vi "PointGrey Grasshopper Temp_Cam.vi"(0 "Operation":T2(ring), 1 "Camera-specific in":variant, 5 "Exposure time (s)":dbl, 7 "Save path":path, 9 "Capture mode":enum16{"Single frame", "Sequence"}(ring), 11 "Capture button":refnum<vi>, 12 "Image in":variant, 14 "Frames in sequence":u32) -> (3 "Camera-specific out":variant, 4 "Status":T1)   [LabVIEW 2015]
uses:
  <vilib>/userdefined/High Color/IMAQdx.ctl
  <vilib>/vision/Image Controls.llb/IMAQ Image.ctl
  <vilib>/vision/driver/IMAQdx.llb/IMAQdx Camera Control Mode.ctl
  <vilib>/vision/driver/IMAQdx.llb/IMAQdx Acquisition Mode.ctl
  <vilib>/Platform/TimedLoop/XDataNode/timing_clust.ctl
  <vilib>/Platform/TimedLoop/XDataNode/nitl_modes.ctl
  <vilib>/Platform/TimedLoop/XDataNode/wakeup.ctl
  <vilib>/vision/driver/IMAQdx.llb/IMAQdx Buffer Number Mode.ctl
  <vilib>/platform/TimedLoop/XDataNode/XDataNode.xnode
  <vilib>/vision/driver/NI_Vision_Acquisition_Software.lvlib
  <resource>/objmgr/imaqdx.rc
  <vilib>/Platform/TimedLoop/XDataNode/XDNodeRunTimeDep.lvlib
  <vilib>/vision/NI_Vision_Development_Module.lvlib
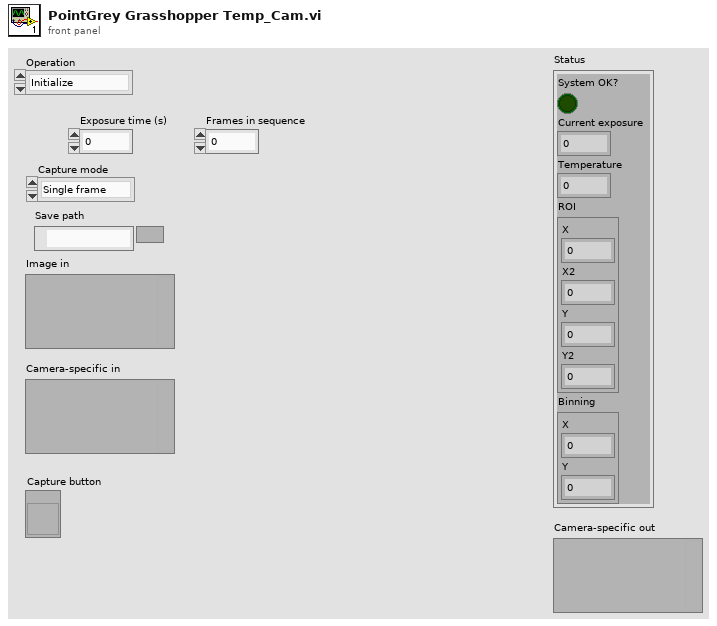
[diagram p1: front panel]
types:
  T1 = cluster{"System OK?":bool, "Current exposure":dbl, "Temperature":dbl, "ROI":cluster{"X":u32, "X2":u32, "Y":u32, "Y2":u32}, "Binning":cluster{"X":u32, "Y":u32}}
  T2 = enum16{"Initialize", "Shut down", "Set capture mode", "Set exposure", "Trigger and read", "Get status", "Other settings"}
  T3 = typedef "IMAQdx.ctl" = refnum<k21>
  T4 = typedef "IMAQ Image.ctl" = refnum<image>
  T5 = typedef "Semaphore RefNum" = refnum<k1>
  T6 = cluster{"Frames to capture":u32, "Current camera":i32, "Camera References":T3[], "Which cameras record":bool[], "Camera event refnums":refnum<event-registration>[], "Image buffers":T4[], "File write access":T5, "Offset and gain":dbl[][], "RGB Channels":enum16{"None", "Camera 1", "Camera 2", "Camera 3"}[], "RGB buffers":T4[], "Camera orientation":enum16{"No rotation, No flip", "No rotation, Flip UD", "No rotation, Flip LR", "Clockwise, No flip", "Clockwise, Flip UD", "Clockwise, Flip LR", "Anticlockwise, No flip", "Anticlockwise, Flip UD", "Anticlockwise, Flip LR"}[]}
  T7 = enum32{"Continuous", "Single frame", "Multi frame"}
  T8 = typedef "NI_Vision_Acquisition_Software.lvlib/IMAQdx Camera Control Mode.ctl" = enum32{"Controller", "Listener"}
  T9 = cluster{"New Image":T4, "Image":refnum<vi>, "FPS target":dbl}
  T10 = enum16{"open", "replace", "create", "open or create", "replace or create", "replace or create with confirmation"}
  T11 = cluster{"File refnum":refnum<file>, "Image File Directory":cluster{cluster{"Field":u16, "Type":u16, "Count":u32, "Value / Offset":u32, "Add IFD Offset?":bool}[], cluster{"Data":u32[], "Add offset?":bool}[]}, "Big endian?":bool, "IFD Offset Size":u32}
  T12 = typedef "NI_Vision_Acquisition_Software.lvlib/IMAQdx Acquisition Mode.ctl" = enum32{"One Shot", "Continuous"}
  T13 = typedef "XDNodeRunTimeDep.lvlib/timing_clust.ctl" = cluster{"Expected End [f-1]":u64, "Actual End [f-1]":u64, "Finished Late? [f-1]":bool, "Expected End [i-1]":u64, "Actual End [i-1]":u64, "Finished Late? [i-1]":bool, "Expected Start [i]":u64, "Actual Start [i]":u64, "Expected Start [f]":u64, "Actual Start [f]":u64, "Source Name":string, "Structure Name":string, "Period":i64, "Deadline":i64, "Offset":i64, "Start":i64, "Priority":i32, "Timeout":i32, "Mode":T14, "Wakeup Reason":T15, "Error":errorcluster, "Source Type":string, "Secondary Source Type":string, "Global End Time":u64, "Global Start Time":u64, "Frame Duration":u64, "Iteration Duration":u64, "Assigned CPU":i32, "I/O Scan Engine Mode":u32}
  T14 = typedef "XDNodeRunTimeDep.lvlib/nitl_modes.ctl" = enum32{"No Change", "Process missed periods, maintain original phase", "Discard missed periods, maintain original phase", "Process missed periods, ignore original phase", "Discard missed periods, ignore original phase"}
  T15 = typedef "XDNodeRunTimeDep.lvlib/wakeup.ctl" = enum32{"Normal", "Aborted", "Asynchronous wakeup", "Timing source error", "Timed loop error", "Timeout"}
  T16 = typedef "NI_Vision_Acquisition_Software.lvlib/IMAQdx Buffer Number Mode.ctl" = enum32{"Next", "Last", "Buffer Number", "Every", "Last New"}
  T17 = typedef "Image Type" = u32
  T18 = enum16{"No rotation, No flip", "No rotation, Flip UD", "No rotation, Flip LR", "Clockwise, No flip", "Clockwise, Flip UD", "Clockwise, Flip LR", "Anticlockwise, No flip", "Anticlockwise, Flip UD", "Anticlockwise, Flip LR"}[]
  T19 = enum16{"None", "Camera 1", "Camera 2", "Camera 3"}[]
  T20 = cluster{"Type":u32, "Version":u32, "Flags":u32, "SerialNumberHigh":u32, "SerialNumberLow":u32, "BusType":u32, "InterfaceName":string, "VendorName":string, "ModelName":string, "CameraFileName":string, "CameraAttributeURL":string}[]
  T21 = enum16{"None", "Camera 1", "Camera 2", "Camera 3"}
  T22 = cluster{"Camera identity":enum16{"Camera 1", "Camera 2", "Camera 3"}, "Timestamp":u64}
  T23 = enum16{"No rotation, No flip", "No rotation, Flip UD", "No rotation, Flip LR", "Clockwise, No flip", "Clockwise, Flip UD", "Clockwise, Flip LR", "Anticlockwise, No flip", "Anticlockwise, Flip UD", "Anticlockwise, Flip LR"}
  T24 = cluster{"element":enum16{"Camera 1", "Camera 2", "Camera 3"}, u64}
  T25 = cluster{"Camera identity":enum16{"Camera 1", "Camera 2", "Camera 3"}, "Timestamp":u64}[]
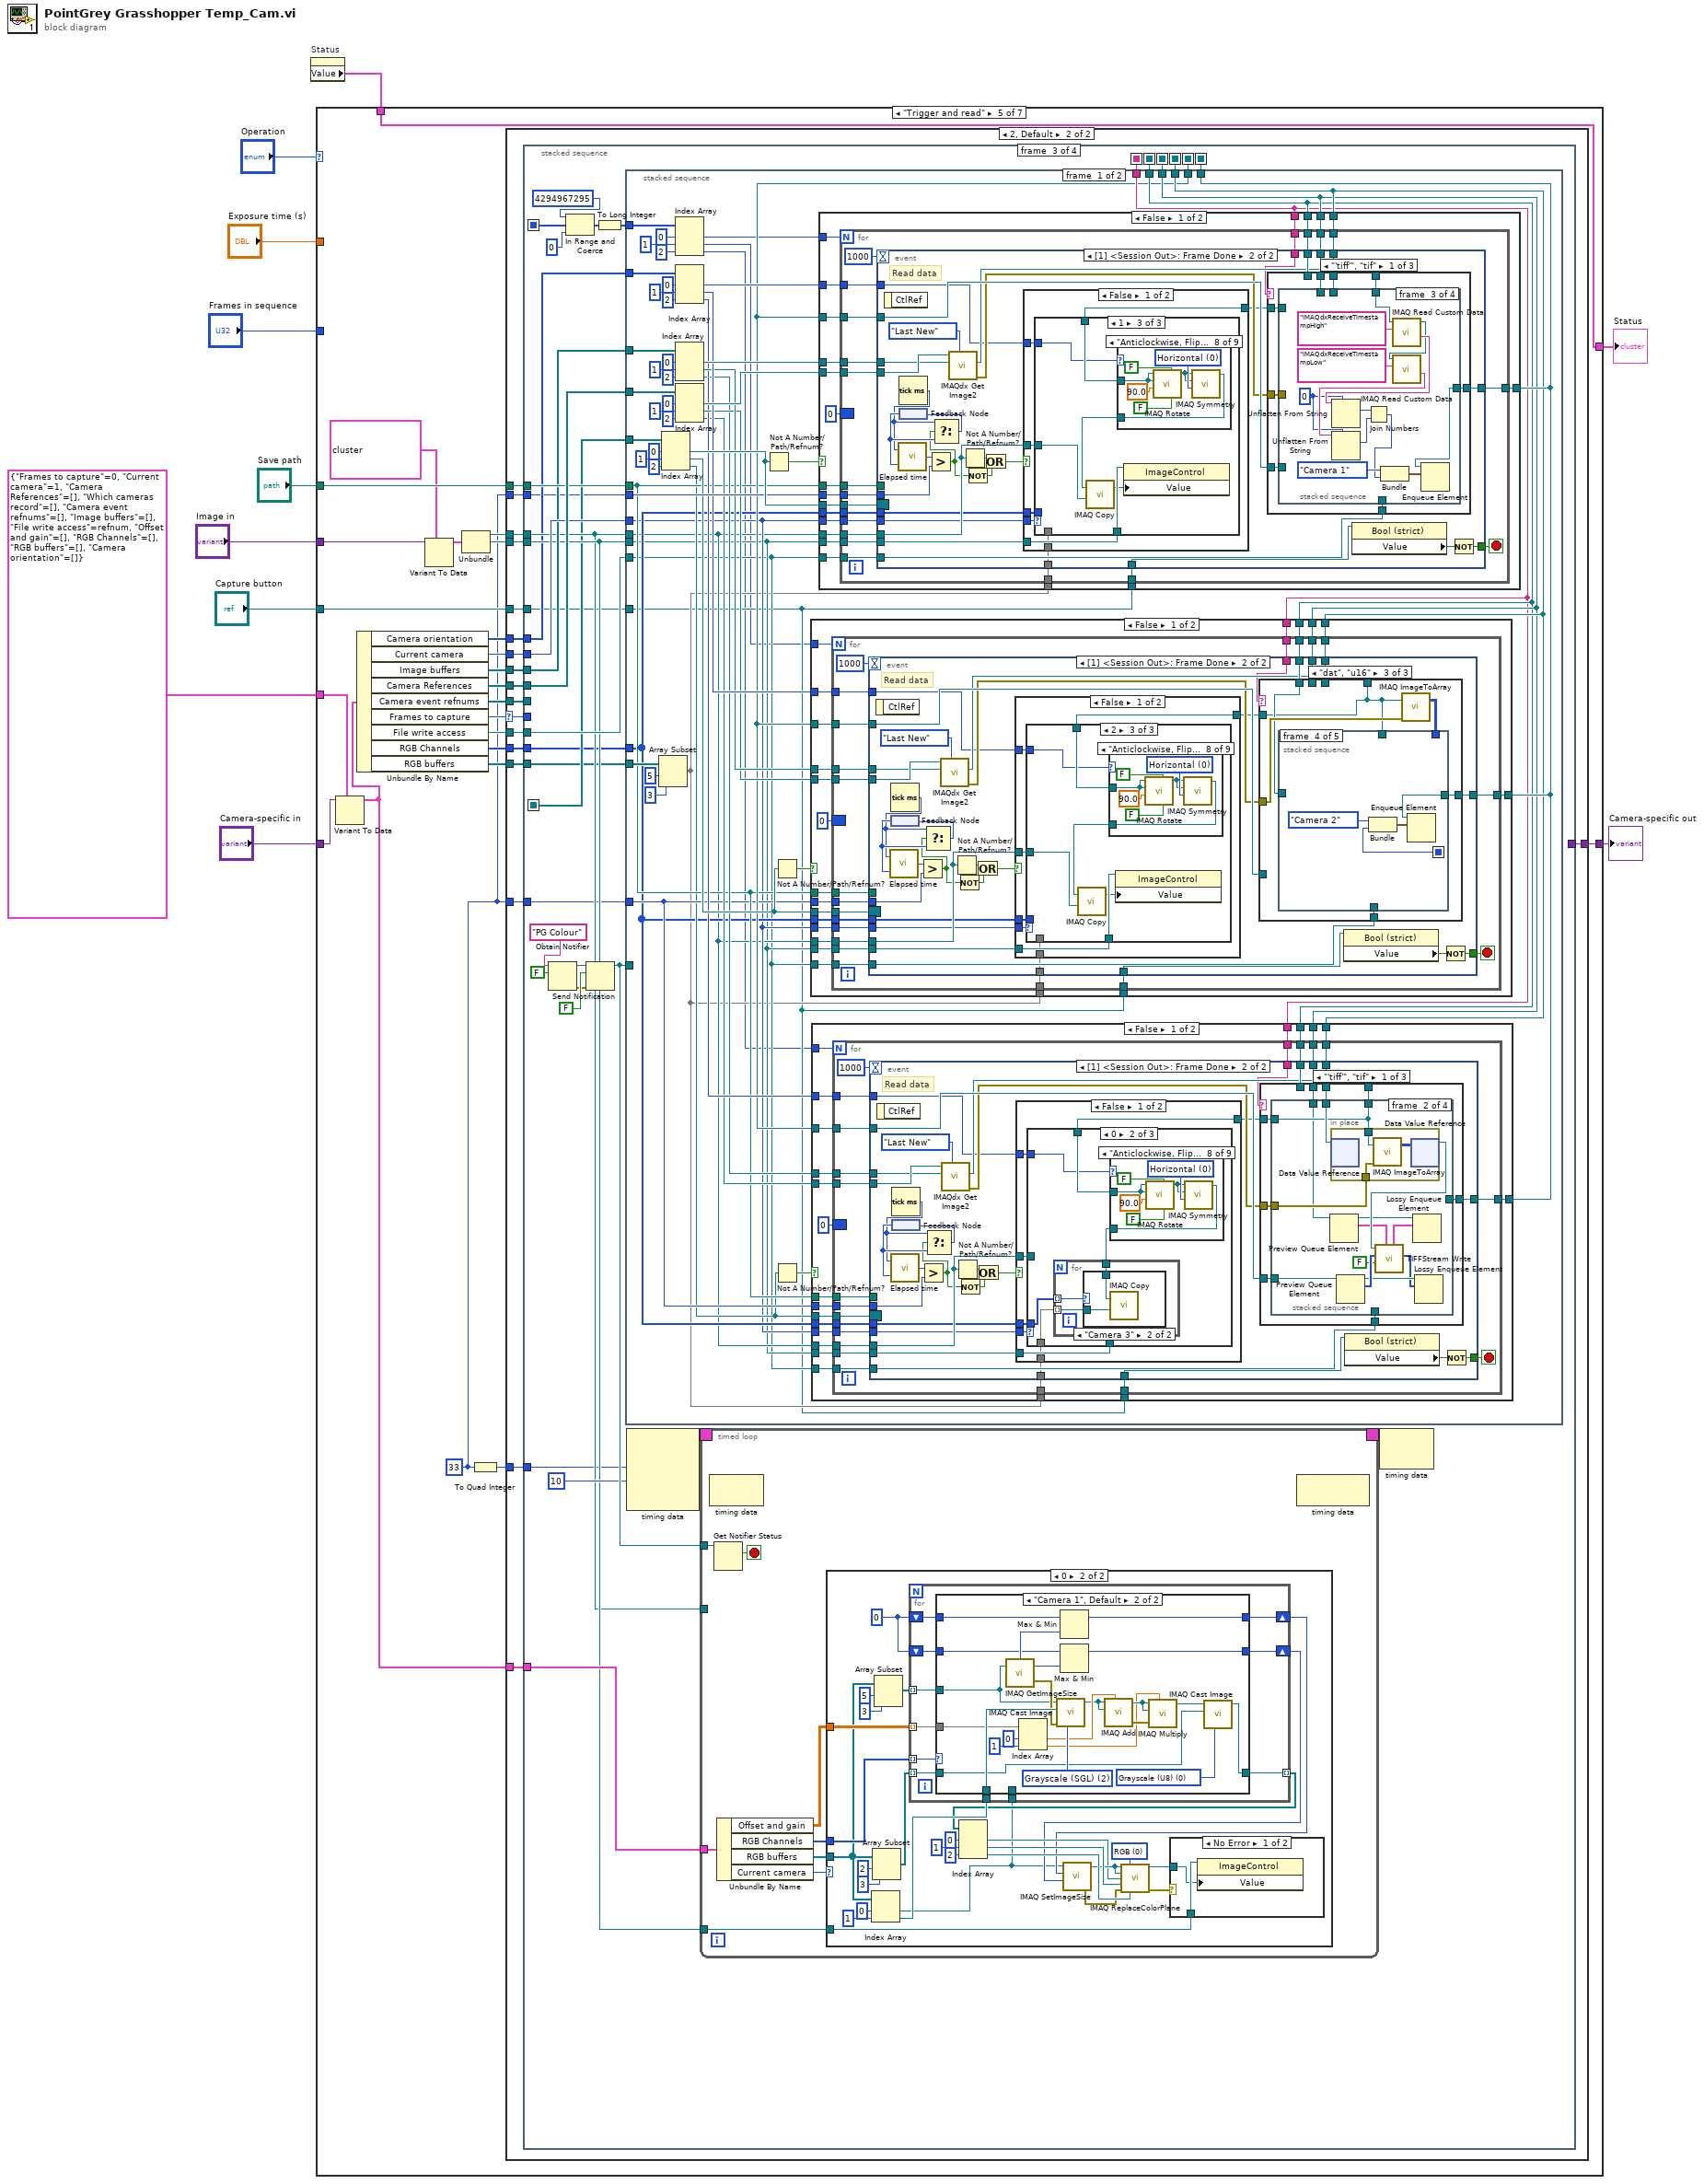
[diagram p0: block diagram]
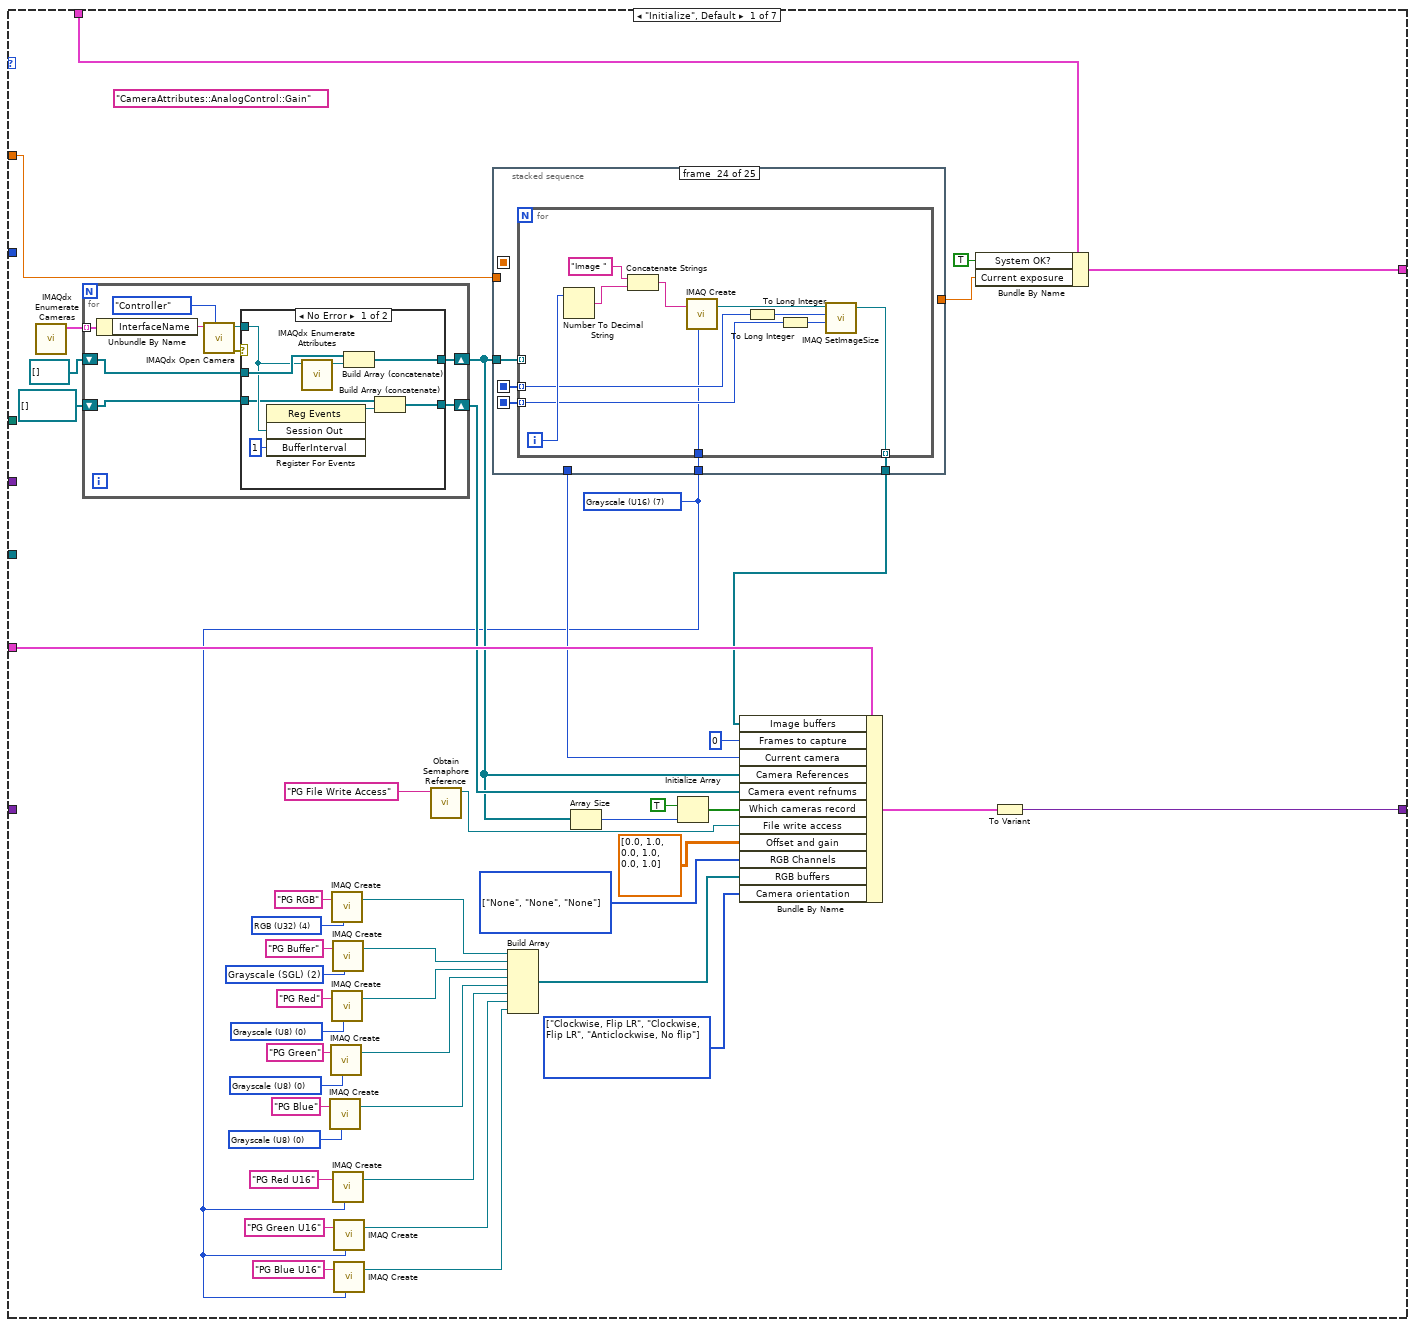
[diagram p2: hidden frame]
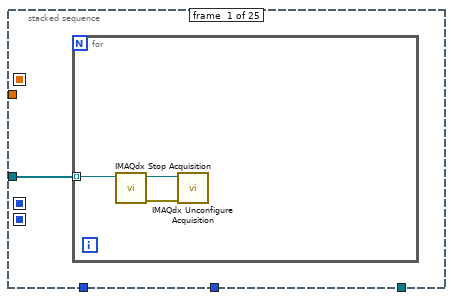
[diagram p3: hidden frame]
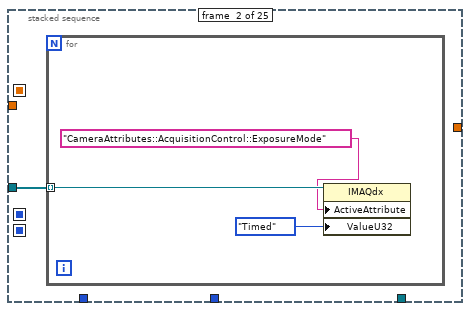
[diagram p4: hidden frame]
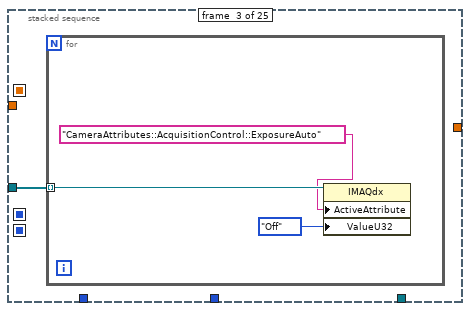
[diagram p5: hidden frame]
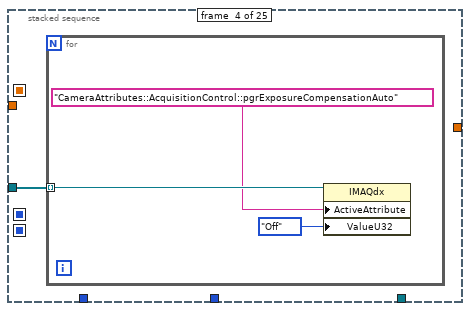
[diagram p6: hidden frame]
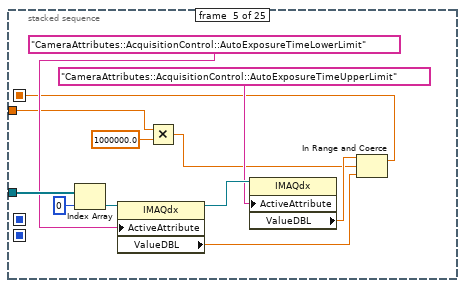
[diagram p7: hidden frame]
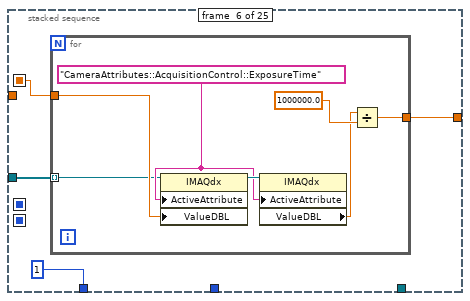
[diagram p8: hidden frame]
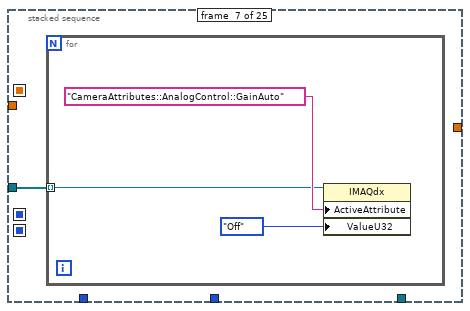
[diagram p9: hidden frame]
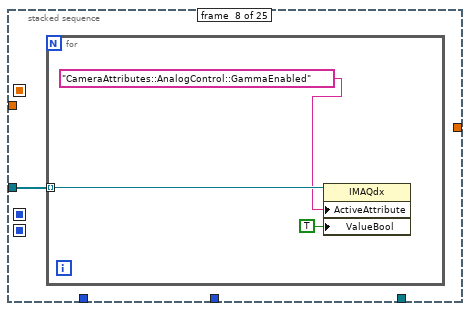
[diagram p10: hidden frame]
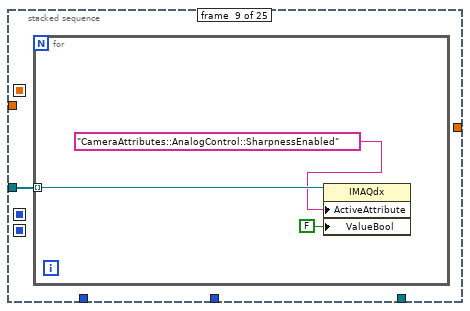
[diagram p11: hidden frame]
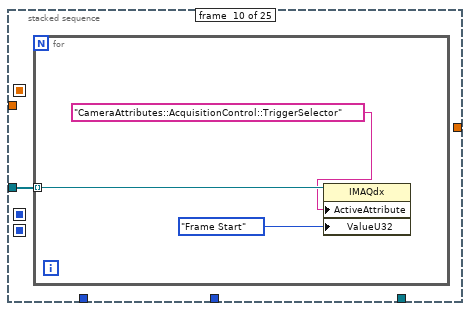
[diagram p12: hidden frame]
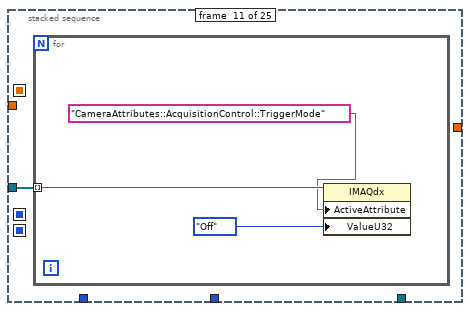
[diagram p13: hidden frame]
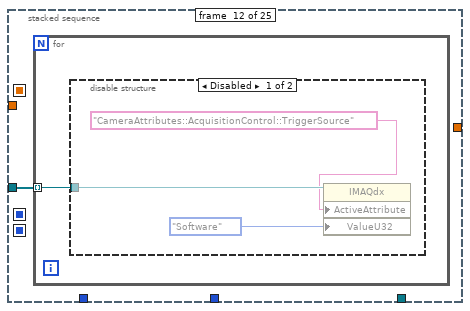
[diagram p14: hidden frame]
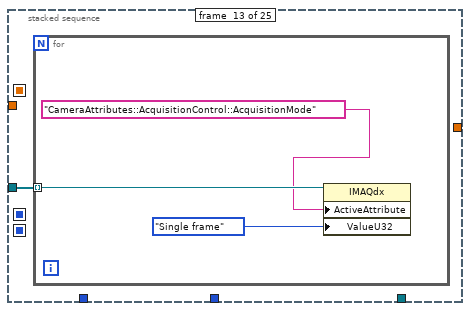
[diagram p16: hidden frame]
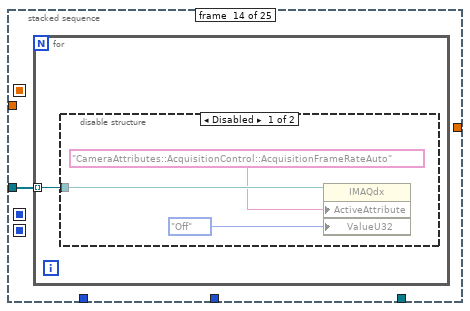
[diagram p17: hidden frame]
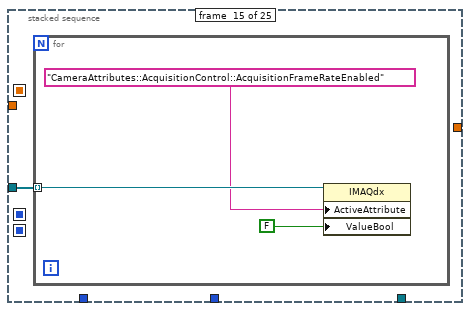
[diagram p19: hidden frame]
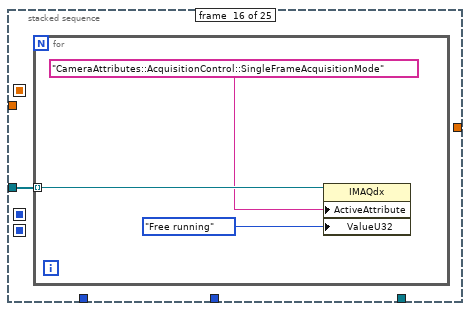
[diagram p20: hidden frame]
diagram:
  n1 = property on="Status" class="Clust (strict)"() -> ("Value"=w9:T1)  [unwired: 2 in, 2 out]
  n2 = case shown="\"Trigger and read\"" "Operation" {
    tunnel: "Exposure time (s)" -> [w47 _ _ w382 _ _ _]
    tunnel: w9 -> [w58 w218 w242 w388 w439 w1791 w1809]
    tunnel: [w57 w218 w242 w387 w439 w1790 w1809] -> w8
    tunnel: "Save path" -> [_ _ _ _ w438 _ _]
    tunnel: "Image in" -> [_ _ _ _ w429 _ _]
    tunnel: [w55 w213 w238 w385 w422 w1787 w1801] -> w5
    tunnel: "Camera-specific in" -> [_ w217 w240 w385 w425 w1787 w1808]
    tunnel: T6 {"Frames to capture"=0, "Current camera"=1, "Camera References"=[], "Which cameras record"=[], "Camera event refnums"=[], "Image buffers"=[], "File write access"=refnum, "Offset and gain"=[], "RGB Channels"=[], "RGB buffers"=[], "Camera orientation"=[]} -> [w56 w212 w239 w386 w437 w1786 w1807]
    tunnel: "Frames in sequence" -> [_ _ w235 _ _ _ _]
    tunnel: "Capture button" -> [_ _ _ _ w421 _ _]
    frame "Initialize", Default {
      w17 = T17 7 items=["Grayscale (U8)", "Grayscale (I16)", "Grayscale (SGL)", "Complex (CSG)", "RGB (U32)", "HSL (U32)", "RGB (U64)", "Grayscale (U16)"] ("Image Type")
      w19 = T18 [enum."Clockwise, Flip LR", enum."Clockwise, Flip LR", enum."Anticlockwise, No flip"] items=["No rotation, No flip", "No rotation, Flip UD", "No rotation, Flip LR", "Clockwise, No flip", "Clockwise, Flip UD", "Clockwise, Flip LR", "Anticlockwise, No flip", "Anticlockwise, Flip UD", "Anticlockwise, Flip LR"] ("Camera orientation")
      w26 = T17 0 items=["Grayscale (U8)", "Grayscale (I16)", "Grayscale (SGL)", "Complex (CSG)", "RGB (U32)", "HSL (U32)", "RGB (U64)", "Grayscale (U16)"] ("Image Type")
      w27 = T17 0 items=["Grayscale (U8)", "Grayscale (I16)", "Grayscale (SGL)", "Complex (CSG)", "RGB (U32)", "HSL (U32)", "RGB (U64)", "Grayscale (U16)"] ("Image Type")
      w28 = T17 0 items=["Grayscale (U8)", "Grayscale (I16)", "Grayscale (SGL)", "Complex (CSG)", "RGB (U32)", "HSL (U32)", "RGB (U64)", "Grayscale (U16)"] ("Image Type")
      w29 = T17 2 items=["Grayscale (U8)", "Grayscale (I16)", "Grayscale (SGL)", "Complex (CSG)", "RGB (U32)", "HSL (U32)", "RGB (U64)", "Grayscale (U16)"] ("Image Type")
      w30 = T17 4 items=["Grayscale (U8)", "Grayscale (I16)", "Grayscale (SGL)", "Complex (CSG)", "RGB (U32)", "HSL (U32)", "RGB (U64)", "Grayscale (U16)"] ("Image Type")
      w36 = T19 [enum."None", enum."None", enum."None"] items=["None", "Camera 1", "Camera 2", "Camera 3"] ("RGB Channels")
      (unwired) "CameraAttributes::AnalogControl::Gain"
      n3 = call <vilib>:"IMAQdx Enumerate Cameras.vi"() -> ("Camera Information Array"=w53:T20)  [unwired: 10 in, 1 out]
      n4 = for {
        tunnel: w53 -> [w198] mode=indexing
        shift-right: [w193] -> w45
        shift-left: T3[] [] -> [w191]
        shift-right: [w194] -> w50
        shift-left: refnum<event-registration>[] [] -> [w190]
        n5 = Unbundle By Name(w198) -> ("InterfaceName"=w197:string)
        n6 = call <vilib>:"IMAQdx Open Camera.vi"("Camera Control Mode"=IMAQdx_Camera_Control_Mode."Controller", "Session In"=w197) -> ("error out"=w192:errorcluster, "Session Out"=w195:T3)  [unwired: 8 in]
        n7 = case shown="No Error" w192 {
          tunnel: w195 -> [w202 _]
          tunnel: [w201 w207] -> w194
          tunnel: [w204 w208] -> w193
          tunnel: w191 -> [w203 w208]
          tunnel: w190 -> [w199 w207]
          frame No Error {
            n8 = register-events(w202, u32 1 ("BufferInterval")) -> (reference out=w200:refnum<event-registration>)  [unwired: 2 in, 1 out]
            n9 = call <vilib>:"IMAQdx Enumerate Attributes.vi"("Session In"=w202) -> ("Session Out"=w205:T3)  [unwired: 8 in, 2 out]
            n10 = Build Array (concatenate)(w203, w205) -> (w204:T3[])
            n11 = Build Array (concatenate)(w199, w200) -> (w201:refnum<event-registration>[])
          }
          frame Error {
          }
        }
      }
      n12 = call "IMAQ Create"("Image Name"="PG Blue", "Image Type"=w26) -> ("New Image"=w21:T4)  [unwired: 3 in, 1 out]
      n13 = call "IMAQ Create"("Image Name"="PG Green", "Image Type"=w27) -> ("New Image"=w22:T4)  [unwired: 3 in, 1 out]
      n14 = call "IMAQ Create"("Image Name"="PG RGB", "Image Type"=w30) -> ("New Image"=w25:T4)  [unwired: 3 in, 1 out]
      n15 = call "IMAQ Create"("Image Name"="PG Red", "Image Type"=w28) -> ("New Image"=w23:T4)  [unwired: 3 in, 1 out]
      n16 = call "IMAQ Create"("Image Name"="PG Buffer", "Image Type"=w29) -> ("New Image"=w24:T4)  [unwired: 3 in, 1 out]
      n17 = call "IMAQ Create"("Image Name"="PG Red U16", "Image Type"=w17) -> ("New Image"=w16:T4)  [unwired: 3 in, 1 out]
      n18 = call "IMAQ Create"("Image Name"="PG Green U16", "Image Type"=w17) -> ("New Image"=w14:T4)  [unwired: 3 in, 1 out]
      n19 = call "IMAQ Create"("Image Name"="PG Blue U16", "Image Type"=w17) -> ("New Image"=w15:T4)  [unwired: 3 in, 1 out]
      n20 = call <vilib>:"Obtain Semaphore Reference.vi"("name (unnamed)"="PG File Write Access") -> ("semaphore"=w38:T5)  [unwired: 4 in, 2 out]
      n21 = stacked-sequence {
        seq-local: [_ _ _ _ w78 _ _ _ _ _ _ _ _ _ _ _ _ _ _ _ _ _ _ _ _] -> [_ _ _ _ _ w87 _ _ _ _ _ _ _ _ _ _ _ _ _ _ _ _ _ _ _]
        seq-local: [_ _ _ _ _ _ _ _ _ _ _ _ _ _ _ _ _ w144 _ _ _ _ _ _ _] -> [_ _ _ _ _ _ _ _ _ _ _ _ _ _ _ _ _ _ _ _ _ _ _ w175 _]
        seq-local: [_ _ _ _ _ _ _ _ _ _ _ _ _ _ _ _ _ _ w150 _ _ _ _ _ _] -> [_ _ _ _ _ _ _ _ _ _ _ _ _ _ _ _ _ _ _ _ _ _ _ w174 _]
        tunnel: w45 -> [w59 w63 w67 w71 w84 w90 w98 w102 w106 w110 w114 w118 w123 w127 w132 w136 w140 w145 w151 w156 w160 w164 w168 w176 w188]
        tunnel: [_ _ _ _ _ 1 ("index") _ _ _ _ _ _ _ _ _ _ _ _ _ _ _ _ _ _ _] -> w48
        tunnel: w47 -> [_ _ _ _ w76 _ _ _ _ _ _ _ _ _ _ _ _ _ _ _ _ _ _ _ _]
        tunnel: [_ _ _ _ _ w88 _ _ _ _ _ _ _ _ _ _ _ _ _ _ _ _ _ _ _] -> w46
        tunnel: [_ _ _ _ _ _ _ _ _ _ _ _ _ _ _ _ _ _ _ _ _ _ _ w173 _] -> w41
        tunnel: w17 -> [_ _ _ _ _ _ _ _ _ _ _ _ _ _ _ _ _ _ _ _ _ _ _ w172 _]
        frame #0 {
          n22 = for {
            tunnel: w59 -> [w62] mode=indexing
            n23 = call <vilib>:"IMAQdx Stop Acquisition.vi"("Session In"=w62) -> ("error out"=w60:errorcluster, "Session Out"=w61:T3)  [unwired: 9 in]
            n24 = call <vilib>:"IMAQdx Unconfigure Acquisition.vi"("error in"=w60, "Session In"=w61) -> ()  [unwired: 8 in, 2 out]
          }
        }
        frame #1 {
          n25 = for {
            tunnel: w63 -> [w66] mode=indexing
            n26 = property class="IMAQdx"(reference=w66, "ActiveAttribute"="CameraAttributes::AcquisitionControl::ExposureMode", "ValueU32"=enum32{"Timed", "Trigger Width"}."Timed") -> ()  [unwired: 1 in, 2 out]
          }
        }
        frame #2 {
          n27 = for {
            tunnel: w67 -> [w70] mode=indexing
            n28 = property class="IMAQdx"(reference=w70, "ActiveAttribute"="CameraAttributes::AcquisitionControl::ExposureAuto", "ValueU32"=enum32{"Off", "Once", "Continuous"}."Off") -> ()  [unwired: 1 in, 2 out]
          }
        }
        frame #3 {
          n29 = for {
            tunnel: w71 -> [w74] mode=indexing
            n30 = property class="IMAQdx"(reference=w74, "ActiveAttribute"="CameraAttributes::AcquisitionControl::pgrExposureCompensationAuto", "ValueU32"=enum32{"Off", "Once", "Continuous"}."Off") -> ()  [unwired: 1 in, 2 out]
          }
        }
        frame #4 {
          n31 = Index Array(array=w84, index=0) -> (element=w86:T3)
          n32 = property class="IMAQdx"(reference=w86, "ActiveAttribute"="CameraAttributes::AcquisitionControl::AutoExposureTimeLowerLimit") -> (reference out=w82:T3, "ValueDBL"=w80:dbl)  [unwired: 1 in, 1 out]
          n33 = Multiply(x=w76, y=1000000.0) -> (x*y=w75:dbl)
          n34 = property class="IMAQdx"(reference=w82, "ActiveAttribute"="CameraAttributes::AcquisitionControl::AutoExposureTimeUpperLimit") -> ("ValueDBL"=w79:dbl)  [unwired: 1 in, 2 out]
          n35 = In Range and Coerce(upper limit=w79, x=w75, lower limit=w80) -> (coerced(x)=w78:dbl)  [unwired: 1 out]
        }
        frame #5 {
          n36 = for {
            tunnel: w90 -> [w91] mode=indexing
            tunnel: [w94] -> w88
            tunnel: w87 -> [w92]
            w93 = "CameraAttributes::AcquisitionControl::ExposureTime"
            n37 = property class="IMAQdx"(reference=w91, "ActiveAttribute"=w93, "ValueDBL"=w92) -> (reference out=w97:T3)  [unwired: 1 in, 1 out]
            n38 = property class="IMAQdx"(reference=w97, "ActiveAttribute"=w93) -> ("ValueDBL"=w95:dbl)  [unwired: 1 in, 2 out]
            n39 = Divide(x=w95, y=1000000.0) -> (x/y=w94:dbl)
          }
        }
        frame #6 {
          n40 = for {
            tunnel: w98 -> [w99] mode=indexing
            n41 = property class="IMAQdx"(reference=w99, "ActiveAttribute"="CameraAttributes::AnalogControl::GainAuto", "ValueU32"=enum32{"Off", "Once", "Continuous"}."Off") -> ()  [unwired: 1 in, 2 out]
          }
        }
        frame #7 {
          n42 = for {
            tunnel: w102 -> [w105] mode=indexing
            n43 = property class="IMAQdx"(reference=w105, "ActiveAttribute"="CameraAttributes::AnalogControl::GammaEnabled", "ValueBool"=TRUE) -> ()  [unwired: 1 in, 2 out]
          }
        }
        frame #8 {
          n44 = for {
            tunnel: w106 -> [w109] mode=indexing
            n45 = property class="IMAQdx"(reference=w109, "ActiveAttribute"="CameraAttributes::AnalogControl::SharpnessEnabled", "ValueBool"=FALSE) -> ()  [unwired: 1 in, 2 out]
          }
        }
        frame #9 {
          n46 = for {
            tunnel: w110 -> [w113] mode=indexing
            n47 = property class="IMAQdx"(reference=w113, "ActiveAttribute"="CameraAttributes::AcquisitionControl::TriggerSelector", "ValueU32"=enum32{"Frame Start", "Exposure Active"}."Frame Start") -> ()  [unwired: 1 in, 2 out]
          }
        }
        frame #10 {
          n48 = for {
            tunnel: w114 -> [w117] mode=indexing
            n49 = property class="IMAQdx"(reference=w117, "ActiveAttribute"="CameraAttributes::AcquisitionControl::TriggerMode", "ValueU32"=enum32{"Off", "On"}."Off") -> ()  [unwired: 1 in, 2 out]
          }
        }
        frame #11 {
          n50 = for {
            tunnel: w118 -> [w119] mode=indexing
            n51 = disable-structure shown="Disabled" {
              disable-tunnel: w119 -> [w122 _]
              frame Disabled {
                n52 = property class="IMAQdx"(reference=w122, "ActiveAttribute"="CameraAttributes::AcquisitionControl::TriggerSource", "ValueU32"=enum32{"Software", "Line 0", "Line 2", "Line 3"}."Software") -> ()  [unwired: 1 in, 2 out]
              }
              frame Enabled {
              }
            }
          }
        }
        frame #12 {
          n53 = for {
            tunnel: w123 -> [w126] mode=indexing
            n54 = property class="IMAQdx"(reference=w126, "ActiveAttribute"="CameraAttributes::AcquisitionControl::AcquisitionMode", "ValueU32"=T7."Single frame") -> ()  [unwired: 1 in, 2 out]
          }
        }
        frame #13 {
          n55 = for {
            tunnel: w127 -> [w128] mode=indexing
            n56 = disable-structure shown="Disabled" {
              disable-tunnel: w128 -> [w131 _]
              frame Disabled {
                n57 = property class="IMAQdx"(reference=w131, "ActiveAttribute"="CameraAttributes::AcquisitionControl::AcquisitionFrameRateAuto", "ValueU32"=enum32{"Off", "Continuous"}."Off") -> ()  [unwired: 1 in, 2 out]
              }
              frame Enabled {
              }
            }
          }
        }
        frame #14 {
          n58 = for {
            tunnel: w132 -> [w135] mode=indexing
            n59 = property class="IMAQdx"(reference=w135, "ActiveAttribute"="CameraAttributes::AcquisitionControl::AcquisitionFrameRateEnabled", "ValueBool"=FALSE) -> ()  [unwired: 1 in, 2 out]
          }
        }
        frame #15 {
          n60 = for {
            tunnel: w136 -> [w139] mode=indexing
            n61 = property class="IMAQdx"(reference=w139, "ActiveAttribute"="CameraAttributes::AcquisitionControl::SingleFrameAcquisitionMode", "ValueU32"=enum16{"Free running", "Triggered"}."Free running") -> ()  [unwired: 1 in, 2 out]
          }
        }
        frame #16 {
          n62 = for {
            tunnel: w140 -> [w143] mode=indexing
            w142 = u32 17563654 items=["Mono 8"=17301505, "Mono 12 Packed (IIDC-msb)"=17563654, "Mono 12 Packed"=17563719, "Mono 16"=17825799]
            n63 = property class="IMAQdx"(reference=w143, "ActiveAttribute"="CameraAttributes::ImageFormatControl::PixelFormat", "ValueU32"=w142) -> ()  [unwired: 1 in, 2 out]
          }
        }
        frame #17 {
          n64 = for {
            tunnel: w145 -> [w149] mode=indexing
            tunnel: [w146] -> w144 mode=indexing
            w148 = "CameraAttributes::ImageFormatControl::Width"
            n65 = property class="IMAQdx"(reference=w149, "ActiveAttribute"=w148) -> (reference out=w147:T3, "MaxU32"=w146:u32)  [unwired: 1 in, 1 out]
            n66 = property class="IMAQdx"(reference=w147, "ActiveAttribute"=w148, "ValueU32"=w146) -> ()  [unwired: 1 in, 2 out]
          }
        }
        frame #18 {
          n67 = for {
            tunnel: w151 -> [w155] mode=indexing
            tunnel: [w152] -> w150 mode=indexing
            w154 = "CameraAttributes::ImageFormatControl::Height"
            n68 = property class="IMAQdx"(reference=w155, "ActiveAttribute"=w154) -> (reference out=w153:T3, "MaxU32"=w152:u32)  [unwired: 1 in, 1 out]
            n69 = property class="IMAQdx"(reference=w153, "ActiveAttribute"=w154, "ValueU32"=w152) -> ()  [unwired: 1 in, 2 out]
          }
        }
        frame #19 {
          n70 = for {
            tunnel: w156 -> [w158] mode=indexing
            n71 = property class="IMAQdx"(reference=w158, "ActiveAttribute"="CameraAttributes::ImageFormatControl::OffsetX", "ValueU32"=u32 0) -> ()  [unwired: 1 in, 2 out]
          }
        }
        frame #20 {
          n72 = for {
            tunnel: w160 -> [w162] mode=indexing
            n73 = property class="IMAQdx"(reference=w162, "ActiveAttribute"="CameraAttributes::ImageFormatControl::OffsetY", "ValueU32"=u32 0) -> ()  [unwired: 1 in, 2 out]
          }
        }
        frame #21 {
          n74 = for {
            tunnel: w164 -> [w166] mode=indexing
            n75 = property class="IMAQdx"(reference=w166, "ActiveAttribute"="CameraAttributes::ImageFormatControl::BinningVertical", "ValueU32"=u32 1) -> ()  [unwired: 1 in, 2 out]
          }
        }
        frame #22 {
          n76 = for {
            tunnel: w168 -> [w170] mode=indexing
            w169 = u16 7 items=["Standard"=0, "2x2 Binning"=1, "2x2 Decimation"=2, "High sensitivity 12-bit ADC"=7]
            n77 = property class="IMAQdx"(reference=w170, "ActiveAttribute"="CameraAttributes::ImageFormatControl::VideoMode", "ValueU32"=w169) -> ()  [unwired: 1 in, 2 out]
          }
        }
        frame #23 {
          n78 = for {
            tunnel: w176 -> [_] mode=indexing
            tunnel: w175 -> [w181] mode=indexing
            tunnel: w174 -> [w180] mode=indexing
            tunnel: [w182] -> w173 mode=indexing
            tunnel: w172 -> [w177]
            i -> [w186]
            n79 = Number To Decimal String(number=w186) -> (decimal integer string=w185:string)  [unwired: 1 in]
            n80 = Concatenate Strings("Image ", w185) -> (w184:string)
            n81 = call "IMAQ Create"("Image Name"=w184, "Image Type"=w177) -> ("New Image"=w183:T4)  [unwired: 3 in, 1 out]
            n82 = To Long Integer(number=w181) -> (32bit integer=w179:i32)
            n83 = To Long Integer(number=w180) -> (32bit integer=w178:i32)
            n84 = call "IMAQ SetImageSize"("Y Resolution"=w178, "X Resolution"=w179, "Image"=w183) -> ("Image Out"=w182:T4)  [unwired: 2 in, 1 out]
          }
        }
        frame #24 {
          n85 = for {
            tunnel: w188 -> [w189] mode=indexing
            n86 = call <vilib>:"IMAQdx Configure Grab.vi"("Session In"=w189) -> ()  [unwired: 9 in, 2 out]
          }
        }
      }
      n87 = Build Array(w25, w24, w23, w22, w21, w16, w14, w15) -> (w20:T4[])
      n88 = Array Size(array=w45) -> (size(s)=w43:i32)
      n89 = Initialize Array(TRUE, w43) -> (w42:bool[])
      n90 = Bundle By Name(cluster=w56, "Image buffers"=w41, "Frames to capture"=u32 0, "Current camera"=w48, "Camera References"=w45, "Camera event refnums"=w50, "Which cameras record"=w42, "File write access"=w38, "Offset and gain"=dbl[][] [[0.0, 1.0], [0.0, 1.0], [0.0, 1.0]], "RGB Channels"=w36, "RGB buffers"=w20, "Camera orientation"=w19) -> (w51:T6)
      n91 = Bundle By Name(cluster=w58, "System OK?"=TRUE, "Current exposure"=w46) -> (w57:T1)
      n92 = To Variant(anything=w51) -> (Variant=w55:variant)
    }
    frame "Shut down" {
      n93 = Variant To Data(type=w212, Variant=w217) -> (data=w216:T6)  [unwired: 1 in, 1 out]
      n94 = Unbundle By Name(w216) -> ("Camera References"=w215:T3[], "Camera event refnums"=w214:refnum<event-registration>[], "File write access"=w211:T5, "Image buffers"=w210:T4[], "RGB buffers"=w209:T4[])
      n95 = for {
        tunnel: w210 -> [w220] mode=indexing
        n96 = call "IMAQ Dispose"("Image"=w220) -> ()  [unwired: 5 in, 1 out]
      }
      n97 = for {
        tunnel: w209 -> [w219] mode=indexing
        n98 = call "IMAQ Dispose"("Image"=w219) -> ()  [unwired: 5 in, 1 out]
      }
      n99 = stacked-sequence {
        tunnel: w215 -> [w221 _]
        tunnel: w214 -> [_ w227]
        frame #0 {
          n100 = for {
            tunnel: w221 -> [w222] mode=indexing
            n101 = call <vilib>:"IMAQdx Stop Acquisition.vi"("Session In"=w222) -> ("error out"=w226:errorcluster, "Session Out"=w225:T3)  [unwired: 9 in]
            n102 = call <vilib>:"IMAQdx Unconfigure Acquisition.vi"("error in"=w226, "Session In"=w225) -> ("error out"=w224:errorcluster, "Session Out"=w223:T3)  [unwired: 8 in]
            n103 = call <vilib>:"IMAQdx Close Camera.vi"("error in"=w224, "Session In"=w223) -> ()  [unwired: 9 in, 1 out]
          }
        }
        frame #1 {
          n104 = for {
            tunnel: w227 -> [w229] mode=indexing
            n105 = Unregister For Events(event registration refnum=w229) -> (error out=w228:errorcluster)  [unwired: 1 in]
            n106 = call <vilib>:"Clear Errors.vi"("error in (no error)"=w228) -> ()  [unwired: 5 in, 2 out]
          }
        }
      }
      n107 = call <vilib>:"Release Semaphore Reference.vi"("semaphore"=w211) -> ()  [unwired: 9 in, 2 out]
      n108 = To Variant(anything=w212) -> (Variant=w213:variant)
    }
    frame "Set capture mode" {
      n109 = Variant To Data(type=w239, Variant=w240) -> (data=w234:T6)  [unwired: 1 in, 1 out]
      n110 = Unbundle By Name(w234) -> ("Camera References"=w233:T3[], "Camera event refnums"=w231:refnum<event-registration>[], "Which cameras record"=w232:bool[])
      n111 = case shown="\"Sequence\"" "Capture mode" {
        tunnel: [w243 w313] -> w236
        tunnel: w235 -> [w244 w314]
        tunnel: w233 -> [w248 w318]
        tunnel: w232 -> [w247 w317]
        tunnel: w231 -> [w246 w316]
        tunnel: [w245 w315] -> w230
        frame "Sequence" {
          n112 = stacked-sequence {
            tunnel: w248 -> [_ w257]
            tunnel: w247 -> [_ w256]
            tunnel: w246 -> [w250 w253]
            tunnel: [_ w255] -> w245
            tunnel: w244 -> [w249 w254]
            tunnel: [w249 _] -> w243
            frame #0 {
              n113 = disable-structure shown="Enabled" {
                disable-tunnel: w250 -> [w251 _]
                frame Disabled {
                  n114 = for {
                    tunnel: w251 -> [w252] mode=indexing
                    n115 = Unregister For Events(event registration refnum=w252) -> ()  [unwired: 1 in, 1 out]
                  }
                }
                frame Enabled {
                }
              }
            }
            frame #1 {
              n116 = for {
                tunnel: w257 -> [w262] mode=indexing
                tunnel: w256 -> [w263] mode=indexing
                shift-right: [w261] -> w255
                shift-left: w253 -> [w260]
                tunnel: w254 -> [w259]
                i -> [w258]
                n117 = case shown="True" w263 {
                  tunnel: w262 -> [_ w267]
                  tunnel: [w264 w268] -> w261
                  tunnel: w260 -> [w264 w269]
                  tunnel: w259 -> [_ w266]
                  tunnel: w258 -> [_ w265]
                  frame False {
                  }
                  frame True {
                    n118 = stacked-sequence {
                      tunnel: w269 -> [_ _ _ _ _ _ _ _ w300 _]
                      tunnel: [_ _ _ _ _ _ _ _ w301 _] -> w268
                      tunnel: w267 -> [w272 w273 w281 w285 w288 w292 w294 w297 w302 w310]
                      tunnel: w266 -> [_ _ w280 _ _ _ _ _ _ _]
                      tunnel: w265 -> [_ _ _ _ _ _ _ _ w299 _]
                      frame #0 {
                        n119 = call <vilib>:"IMAQdx Stop Acquisition.vi"("Session In"=w272) -> ("error out"=w270:errorcluster, "Session Out"=w271:T3)  [unwired: 9 in]
                        n120 = call <vilib>:"IMAQdx Unconfigure Acquisition.vi"("error in"=w270, "Session In"=w271) -> ()  [unwired: 8 in, 2 out]
                      }
                      frame #1 {
                        n121 = disable-structure shown="Enabled" {
                          disable-tunnel: w273 -> [w274 w277]
                          frame Disabled {
                            n122 = property class="IMAQdx"(reference=w274, "ActiveAttribute"="CameraAttributes::AcquisitionControl::AcquisitionMode", "ValueU32"=T7."Multi frame") -> ()  [unwired: 1 in, 2 out]
                          }
                          frame Enabled {
                            n123 = property class="IMAQdx"(reference=w277, "ActiveAttribute"="CameraAttributes::AcquisitionControl::AcquisitionMode", "ValueU32"=T7."Continuous") -> ()  [unwired: 1 in, 2 out]
                          }
                        }
                      }
                      frame #2 {
                        n124 = disable-structure shown="Enabled" {
                          disable-tunnel: w281 -> [w283 _]
                          disable-tunnel: w280 -> [w282 _]
                          frame Disabled {
                            n125 = property class="IMAQdx"(reference=w283, "ActiveAttribute"="CameraAttributes::AcquisitionControl::AcquisitionFrameCount", "ValueU32"=w282) -> ()  [unwired: 1 in, 2 out]
                          }
                          frame Enabled {
                          }
                        }
                      }
                      frame #3 {
                        n126 = property class="IMAQdx"(reference=w285, "ActiveAttribute"="CameraAttributes::AcquisitionControl::TriggerSource", "ValueU32"=enum32{"Software", "Line 0", "Line 2", "Line 3"}."Software") -> ()  [unwired: 1 in, 2 out]
                      }
                      frame #4 {
                        n127 = property class="IMAQdx"(reference=w288, "ActiveAttribute"="CameraAttributes::AcquisitionControl::TriggerSelector", "ValueU32"=enum32{"Frame Start", "Exposure Active"}."Frame Start") -> ()  [unwired: 1 in, 2 out]
                      }
                      frame #5 {
                        n128 = property class="IMAQdx"(reference=w292, "ActiveAttribute"="CameraAttributes::AcquisitionControl::TriggerMode", "ValueU32"=enum32{"Off", "On"}."Off") -> ()  [unwired: 1 in, 2 out]
                      }
                      frame #6 {
                        n129 = property class="IMAQdx"(reference=w294, "ActiveAttribute"="CameraAttributes::AcquisitionControl::SingleFrameAcquisitionMode", "ValueU32"=enum16{"Free running", "Triggered"}."Triggered") -> ()  [unwired: 1 in, 2 out]
                      }
                      frame #7 {
                        n130 = disable-structure shown="Enabled" {
                          disable-tunnel: w297 -> [w298 _]
                          frame Disabled {
                            n131 = call <vilib>:"IMAQdx Configure Grab.vi"("Session In"=w298) -> ()  [unwired: 9 in, 2 out]
                          }
                          frame Enabled {
                          }
                        }
                      }
                      frame #8 {
                        n132 = disable-structure shown="Enabled" {
                          disable-tunnel: w302 -> [w308 _]
                          disable-tunnel: [w306 w309] -> w301
                          disable-tunnel: w300 -> [w305 w309]
                          disable-tunnel: w299 -> [w303 _]
                          frame Disabled {
                            n133 = register-events(w308, u32 1 ("BufferInterval")) -> (reference out=w304:refnum<event-registration>)  [unwired: 2 in, 1 out]
                            n134 = Replace Array Subset(array=w305, new element=w304, index=w303) -> (w306:refnum<event-registration>[])
                          }
                          frame Enabled {
                          }
                        }
                      }
                      frame #9 {
                        n135 = property class="IMAQdx"(reference=w310, "ActiveAttribute"="AcquisitionAttributes::ReceiveTimestampMode", "ValueU32"=enum16{"None", "Tick count", "System time"}."System time") -> ()  [unwired: 1 in, 2 out]
                      }
                    }
                  }
                }
              }
            }
          }
        }
        frame "Single frame", Default {
          n136 = stacked-sequence {
            tunnel: w318 -> [_ w327]
            tunnel: w317 -> [_ w326]
            tunnel: w316 -> [w320 w323]
            tunnel: [_ w325] -> w315
            tunnel: w314 -> [_ w324]
            tunnel: [u32 0 ("Frames in sequence") _] -> w313
            frame #0 {
              n137 = disable-structure shown="Enabled" {
                disable-tunnel: w320 -> [w321 _]
                frame Disabled {
                  n138 = for {
                    tunnel: w321 -> [w322] mode=indexing
                    n139 = Unregister For Events(event registration refnum=w322) -> ()  [unwired: 1 in, 1 out]
                  }
                }
                frame Enabled {
                }
              }
            }
            frame #1 {
              n140 = for {
                tunnel: w327 -> [w332] mode=indexing
                tunnel: w326 -> [w333] mode=indexing
                shift-right: [w331] -> w325
                shift-left: w323 -> [w330]
                tunnel: w324 -> [w329]
                i -> [w328]
                n141 = case shown="True" w333 {
                  tunnel: w332 -> [_ w337]
                  tunnel: [w334 w338] -> w331
                  tunnel: w330 -> [w334 w339]
                  tunnel: w329 -> [_ w336]
                  tunnel: w328 -> [_ w335]
                  frame False {
                  }
                  frame True {
                    n142 = stacked-sequence {
                      tunnel: w339 -> [_ w344 _ _ _ _ _ _ _]
                      tunnel: [_ w345 _ _ _ _ _ _ _] -> w338
                      tunnel: w337 -> [w342 w346 w354 w362 w366 w369 w373 w375 w378]
                      tunnel: w336 -> [_ _ _ w361 _ _ _ _ _]
                      tunnel: w335 -> [_ w343 _ _ _ _ _ _ _]
                      frame #0 {
                        n143 = call <vilib>:"IMAQdx Stop Acquisition.vi"("Session In"=w342) -> ("error out"=w340:errorcluster, "Session Out"=w341:T3)  [unwired: 9 in]
                        n144 = call <vilib>:"IMAQdx Unconfigure Acquisition.vi"("error in"=w340, "Session In"=w341) -> ()  [unwired: 8 in, 2 out]
                      }
                      frame #1 {
                        n145 = disable-structure shown="Enabled" {
                          disable-tunnel: w346 -> [w352 _]
                          disable-tunnel: [w350 w353] -> w345
                          disable-tunnel: w344 -> [w349 w353]
                          disable-tunnel: w343 -> [w347 _]
                          frame Disabled {
                            n146 = register-events(w352, u32 1 ("BufferInterval")) -> (reference out=w348:refnum<event-registration>)  [unwired: 2 in, 1 out]
                            n147 = Replace Array Subset(array=w349, new element=w348, index=w347) -> (w350:refnum<event-registration>[])
                          }
                          frame Enabled {
                          }
                        }
                      }
                      frame #2 {
                        n148 = disable-structure shown="Enabled" {
                          disable-tunnel: w354 -> [w355 w358]
                          frame Disabled {
                            n149 = property class="IMAQdx"(reference=w355, "ActiveAttribute"="CameraAttributes::AcquisitionControl::AcquisitionMode", "ValueU32"=T7."Multi frame") -> ()  [unwired: 1 in, 2 out]
                          }
                          frame Enabled {
                            n150 = property class="IMAQdx"(reference=w358, "ActiveAttribute"="CameraAttributes::AcquisitionControl::AcquisitionMode", "ValueU32"=T7."Continuous") -> ()  [unwired: 1 in, 2 out]
                          }
                        }
                      }
                      frame #3 {
                        n151 = disable-structure shown="Enabled" {
                          disable-tunnel: w362 -> [w364 _]
                          disable-tunnel: w361 -> [w363 _]
                          frame Disabled {
                            n152 = property class="IMAQdx"(reference=w364, "ActiveAttribute"="CameraAttributes::AcquisitionControl::AcquisitionFrameCount", "ValueU32"=w363) -> ()  [unwired: 1 in, 2 out]
                          }
                          frame Enabled {
                          }
                        }
                      }
                      frame #4 {
                        n153 = property class="IMAQdx"(reference=w366, "ActiveAttribute"="CameraAttributes::AcquisitionControl::TriggerSource", "ValueU32"=enum32{"Software", "Line 0", "Line 2", "Line 3"}."Software") -> ()  [unwired: 1 in, 2 out]
                      }
                      frame #5 {
                        n154 = property class="IMAQdx"(reference=w369, "ActiveAttribute"="CameraAttributes::AcquisitionControl::TriggerSelector", "ValueU32"=enum32{"Frame Start", "Exposure Active"}."Frame Start") -> ()  [unwired: 1 in, 2 out]
                      }
                      frame #6 {
                        n155 = property class="IMAQdx"(reference=w373, "ActiveAttribute"="CameraAttributes::AcquisitionControl::TriggerMode", "ValueU32"=enum32{"Off", "On"}."Off") -> ()  [unwired: 1 in, 2 out]
                      }
                      frame #7 {
                        n156 = property class="IMAQdx"(reference=w375, "ActiveAttribute"="CameraAttributes::AcquisitionControl::SingleFrameAcquisitionMode", "ValueU32"=enum16{"Free running", "Triggered"}."Triggered") -> ()  [unwired: 1 in, 2 out]
                      }
                      frame #8 {
                        n157 = disable-structure shown="Enabled" {
                          disable-tunnel: w378 -> [w379 _]
                          frame Disabled {
                            n158 = call <vilib>:"IMAQdx Configure Grab.vi"("Session In"=w379) -> ()  [unwired: 9 in, 2 out]
                          }
                          frame Enabled {
                          }
                        }
                      }
                    }
                  }
                }
              }
            }
          }
        }
      }
      n159 = Bundle By Name(cluster=w234, "Frames to capture"=w236, "Camera event refnums"=w230) -> (w237:T6)
      n160 = To Variant(anything=w237) -> (Variant=w238:variant)
    }
    frame "Set exposure" {
      n161 = Variant To Data(type=w386, Variant=w385) -> (data=w384:T6)  [unwired: 1 in, 1 out]
      n162 = Unbundle By Name(w384) -> ("Camera References"=w381:T3[], "Current camera"=w380:i32)
      n163 = case shown="1, Default" w380 {
        selector: w380 -> [_ w391]
        tunnel: [w389 w394] -> w383
        tunnel: w382 -> [w389 w393]
        tunnel: w381 -> [_ w392]
        frame 65535 {
        }
        frame 1, Default {
          n164 = Decrement(x=w391) -> (x-1=w390:i32)
          n165 = stacked-sequence {
            seq-local: [w399 _] -> [_ w408]
            tunnel: w392 -> [w405 w407]
            tunnel: w393 -> [w397 _]
            tunnel: [_ w409] -> w394
            tunnel: w390 -> [_ _]
            frame #0 {
              n166 = Index Array(array=w405, index=0) -> (element=w406:T3)
              n167 = property class="IMAQdx"(reference=w406, "ActiveAttribute"="CameraAttributes::AcquisitionControl::AutoExposureTimeLowerLimit") -> (reference out=w403:T3, "ValueDBL"=w401:dbl)  [unwired: 1 in, 1 out]
              n168 = Multiply(x=w397, y=1000000.0) -> (x*y=w396:dbl)
              n169 = property class="IMAQdx"(reference=w403, "ActiveAttribute"="CameraAttributes::AcquisitionControl::AutoExposureTimeUpperLimit") -> ("ValueDBL"=w400:dbl)  [unwired: 1 in, 2 out]
              n170 = In Range and Coerce(upper limit=w400, x=w396, lower limit=w401) -> (coerced(x)=w399:dbl)  [unwired: 1 out]
            }
            frame #1 {
              n171 = for {
                tunnel: [w413] -> w409
                tunnel: w408 -> [w411]
                tunnel: w407 -> [w410] mode=indexing
                w412 = "CameraAttributes::AcquisitionControl::ExposureTime"
                n172 = property class="IMAQdx"(reference=w410, "ActiveAttribute"=w412, "ValueDBL"=w411) -> (reference out=w416:T3)  [unwired: 1 in, 1 out]
                n173 = property class="IMAQdx"(reference=w416, "ActiveAttribute"=w412) -> ("ValueDBL"=w414:dbl)  [unwired: 1 in, 2 out]
                n174 = Divide(x=w414, y=1000000.0) -> (x/y=w413:dbl)
              }
            }
          }
        }
      }
      n175 = Bundle By Name(cluster=w388, "Current exposure"=w383) -> (w387:T1)
    }
    frame "Trigger and read" {
      w418 = u32 33 ("Period")
      n176 = Variant To Data(type=w437, Variant=w425) -> (data=w424:T6)  [unwired: 1 in, 1 out]
      n177 = Unbundle By Name(w424) -> ("Camera orientation"=w423:T18, "Current camera"=w432:i32, "Image buffers"=w433:T4[], "Camera References"=w435:T3[], "Camera event refnums"=w434:refnum<event-registration>[], "Frames to capture"=w436:u32, "File write access"=w426:T5, "RGB Channels"=w420:T19, "RGB buffers"=w419:T4[])
      n178 = Variant To Data(type=T9 {"New Image"=refnum, "Image"=refnum, "FPS target"=30.0} ("output cluster"), Variant=w429) -> (data=w431:T9)  [unwired: 1 in, 1 out]
      n179 = Unbundle(w431) -> ("New Image"=w428:T4, "Image"=w427:refnum<vi>)  [unwired: 1 out]
      n180 = To Quad Integer(1:w418) -> (0:w417:i64)
      n181 = case shown="2, Default" w436 {
        selector: w436 -> [_ w637]
        tunnel: w438 -> [w444 w643]
        tunnel: w428 -> [w445 w642]
        tunnel: w435 -> [w448 w641]
        tunnel: w434 -> [_ w640]
        tunnel: w433 -> [w447 w639]
        tunnel: w432 -> [w446 w638]
        tunnel: w427 -> [w443 w636]
        tunnel: w426 -> [_ w635]
        tunnel: w424 -> [w441 w634]
        tunnel: w423 -> [w442 w633]
        tunnel: [w440 w632] -> w422
        tunnel: w421 -> [_ w631]
        tunnel: w420 -> [_ w630]
        tunnel: w419 -> [_ w629]
        tunnel: w418 -> [_ w628]
        tunnel: w417 -> [_ w627]
        tunnel: w418 -> [_ w626]
        frame 0 {
          n182 = stacked-sequence {
            tunnel: w448 -> [w455 _]
            tunnel: w447 -> [w453 w547]
            tunnel: w446 -> [w452 _]
            tunnel: w445 -> [w451 w544]
            tunnel: w444 -> [w450 _]
            tunnel: w441 -> [_ w546]
            tunnel: w443 -> [_ w545]
            tunnel: w442 -> [w449 _]
            frame #0 {
              n183 = Array Size(array=w453) -> (size(s)=w454:i32)
              n184 = for {
                tunnel: w453 -> [w468] mode=indexing
                tunnel: w455 -> [w469] mode=indexing
                workers-P: w454 -> [_]
                tunnel: w452 -> [w467]
                tunnel: w451 -> [w464]
                tunnel: w450 -> [w460]
                tunnel: w449 -> [w456] mode=indexing
                i -> [w466]
                n185 = Decrement(x=w467) -> (x-1=w459:i32)
                n186 = Equal?(x=w459, y=w466) -> (x = y?=w465:bool)
                n187 = call <vilib>:"IMAQdx Snap2.vi"("Image In"=w468, "Session In"=w469) -> ("Image Out"=w458:T4)  [unwired: 7 in, 2 out]
                n188 = case shown="\"Clockwise, Flip LR\"" w456 {
                  tunnel: w458 -> [w470 w473 w476 w479 w486 w493 w496 w505 w512]
                  tunnel: [w470 w472 w475 w477 w482 w489 w497 w501 w508] -> w457
                  frame "No rotation, No flip", Default {
                  }
                  frame "No rotation, Flip UD" {
                    w471 = u32 0 items=["Horizontal", "Vertical", "Central", "1st Diagonal", "2nd Diagonal"] ("Type of Symmetry")
                    n189 = call "IMAQ Symmetry"("Type of Symmetry"=w471, "Image Dst"=w473, "Image Src"=w473) -> ("Image Dst Out"=w472:T4)  [unwired: 2 in, 1 out]
                  }
                  frame "No rotation, Flip LR" {
                    w474 = u32 1 items=["Horizontal", "Vertical", "Central", "1st Diagonal", "2nd Diagonal"] ("Type of Symmetry")
                    n190 = call "IMAQ Symmetry"("Type of Symmetry"=w474, "Image Dst"=w476, "Image Src"=w476) -> ("Image Dst Out"=w475:T4)  [unwired: 2 in, 1 out]
                  }
                  frame "Clockwise, No flip" {
                    n191 = call "IMAQ Rotate"("Use Bilinear Interpolation"=FALSE, "Maintain Size"=FALSE, "Angle (degrees)"=sgl 270.0, "Image Dst"=w479, "Image Src"=w479) -> ("Image Dst Out"=w477:T4)  [unwired: 5 in, 1 out]
                  }
                  frame "Clockwise, Flip UD" {
                    w484 = u32 0 items=["Horizontal", "Vertical", "Central", "1st Diagonal", "2nd Diagonal"] ("Type of Symmetry")
                    n192 = call "IMAQ Rotate"("Use Bilinear Interpolation"=FALSE, "Maintain Size"=FALSE, "Angle (degrees)"=sgl 270.0, "Image Dst"=w486, "Image Src"=w486) -> ("Image Dst Out"=w483:T4)  [unwired: 5 in, 1 out]
                    n193 = call "IMAQ Symmetry"("Type of Symmetry"=w484, "Image Dst"=w483, "Image Src"=w483) -> ("Image Dst Out"=w482:T4)  [unwired: 2 in, 1 out]
                  }
                  frame "Clockwise, Flip LR" {
                    w491 = u32 1 items=["Horizontal", "Vertical", "Central", "1st Diagonal", "2nd Diagonal"] ("Type of Symmetry")
                    n194 = call "IMAQ Rotate"("Use Bilinear Interpolation"=FALSE, "Maintain Size"=FALSE, "Angle (degrees)"=sgl 270.0, "Image Dst"=w493, "Image Src"=w493) -> ("Image Dst Out"=w490:T4)  [unwired: 5 in, 1 out]
                    n195 = call "IMAQ Symmetry"("Type of Symmetry"=w491, "Image Dst"=w490, "Image Src"=w490) -> ("Image Dst Out"=w489:T4)  [unwired: 2 in, 1 out]
                  }
                  frame "Anticlockwise, No flip" {
                    n196 = call "IMAQ Rotate"("Use Bilinear Interpolation"=FALSE, "Maintain Size"=FALSE, "Angle (degrees)"=sgl 90.0, "Image Dst"=w496, "Image Src"=w496) -> ("Image Dst Out"=w497:T4)  [unwired: 5 in, 1 out]
                  }
                  frame "Anticlockwise, Flip UD" {
                    w503 = u32 0 items=["Horizontal", "Vertical", "Central", "1st Diagonal", "2nd Diagonal"] ("Type of Symmetry")
                    n197 = call "IMAQ Rotate"("Use Bilinear Interpolation"=FALSE, "Maintain Size"=FALSE, "Angle (degrees)"=sgl 90.0, "Image Dst"=w505, "Image Src"=w505) -> ("Image Dst Out"=w502:T4)  [unwired: 5 in, 1 out]
                    n198 = call "IMAQ Symmetry"("Type of Symmetry"=w503, "Image Dst"=w502, "Image Src"=w502) -> ("Image Dst Out"=w501:T4)  [unwired: 2 in, 1 out]
                  }
                  frame "Anticlockwise, Flip LR" {
                    w510 = u32 1 items=["Horizontal", "Vertical", "Central", "1st Diagonal", "2nd Diagonal"] ("Type of Symmetry")
                    n199 = call "IMAQ Rotate"("Use Bilinear Interpolation"=FALSE, "Maintain Size"=FALSE, "Angle (degrees)"=sgl 90.0, "Image Dst"=w512, "Image Src"=w512) -> ("Image Dst Out"=w509:T4)  [unwired: 5 in, 1 out]
                    n200 = call "IMAQ Symmetry"("Type of Symmetry"=w510, "Image Dst"=w509, "Image Src"=w509) -> ("Image Dst Out"=w508:T4)  [unwired: 2 in, 1 out]
                  }
                }
                n201 = case shown="True" w465 {
                  tunnel: w457 -> [_ w542]
                  tunnel: w464 -> [_ w543]
                  frame False {
                  }
                  frame True {
                    n202 = call "IMAQ Copy"("Image Dst"=w543, "Image Src"=w542) -> ()  [unwired: 4 in, 2 out]
                  }
                }
                n203 = call "IMAQ GetImageSize"("Image"=w457) -> ("Y Resolution"=w461:i32, "X Resolution"=w462:i32)  [unwired: 3 in, 1 out]
                n204 = Not A Number/Path/Refnum?(number/path/refnum=w460) -> (NaN/Path/Refnum?=w463:bool)
                n205 = case shown="False" w463 {
                  tunnel: w460 -> [w518 _]
                  tunnel: w457 -> [w519 _]
                  tunnel: w462 -> [w516 _]
                  tunnel: w461 -> [w515 _]
                  frame False {
                    n206 = call <vilib>:"Get File Extension.vi"("file"=w518) -> ("lowercase file extension"=w517:string)  [unwired: 6 in, 4 out]
                    n207 = case shown="\"dat\", \"u16\"" w517 {
                      tunnel: w518 -> [w532 w541 _]
                      tunnel: w519 -> [w522 w536 _]
                      tunnel: w516 -> [w530 _ _]
                      tunnel: w515 -> [w529 _ _]
                      frame "'tiff'", "tif" {
                        n208 = call "TIFFStream Open.vi"("Bytes per strip"=u32 8000, "File path"=w532, "Height Pixels"=w529, "Width Pixels"=w530, "Big endian?"=FALSE) -> ("error out"=w526:errorcluster, "Current and next IFD offset"=w524:u32[], "Image data reference"=w523:refnum<data-value>, "File data"=w528:T11)  [unwired: 3 in]
                        n209 = in-place {
                          in-place-border: w522 -> [w534]
                          n210 = in-place-dvr #1(w523) -> ()  [unwired: 2 out]
                          n211 = call "IMAQ ImageToArray"("Image"=w534) -> ("Image Pixels (I16)"=w533:i16[][])  [unwired: 3 in, 4 out]
                          n212 = in-place-dvr #1(w533) -> (w520:refnum<data-value>)  [unwired: 1 out]
                        }
                        n213 = call "TIFFStream Write.vi"("File data"=w528, "error in (no error)"=w526, "Last image in file?"=TRUE, "Current and next IFD offset in"=w524, "Image data reference"=w520) -> ("error out"=w527:errorcluster)  [unwired: 4 in, 2 out]
                        n214 = call "TIFFStream Close.vi"("error in (no error)"=w527, "Image data reference"=w520, "File data"=w528) -> ()  [unwired: 8 in, 1 out]
                      }
                      frame "dat", "u16" {
                        # "No need to cast - no negative values"
                        n215 = Open/Create/Replace File(file path (use dialog)=w541, operation (0:open)=T10."replace or create") -> (refnum out=w540:refnum<file>)  [unwired: 4 in, 2 out]
                        n216 = call "IMAQ ImageToArray"("Image"=w536) -> ("Image Pixels (I16)"=w535:i16[][])  [unwired: 3 in, 4 out]
                        n217 = Write to Binary File(file (use dialog)=w540, data=w535, 5:FALSE ("prepend array or string size? (T)")) -> (refnum out=w538:refnum<file>)  [unwired: 3 in, 2 out]
                        n218 = Close File(refnum=w538) -> ()  [unwired: 1 in, 2 out]
                      }
                      frame "None", Default {
                      }
                    }
                  }
                  frame True {
                  }
                }
              }
            }
            frame #1 {
              n219 = Unbundle By Name(w546) -> ("Offset and gain"=w551:dbl[][], "RGB Channels"=w550:T19, "RGB buffers"=w549:T4[], "Current camera"=w548:i32)
              n220 = case shown="0" w548 {
                tunnel: w551 -> [_ w576]
                tunnel: w550 -> [_ w575]
                tunnel: w547 -> [_ w574]
                tunnel: w549 -> [_ w572]
                tunnel: w545 -> [_ w570]
                tunnel: w544 -> [_ w556]
                frame 1, Default {
                }
                frame 0 {
                  w555 = 0 ("X Resolution")
                  w561 = u16 0 items=["RGB", "HSL", "HSV", "HSI"] ("Color Mode")
                  n221 = Index Array(array=w572, index #1=0 ("index"), index #2=1 ("index")) -> (element #1=w552:T4, element #2=w568:T4)
                  n222 = Array Subset(array=w572, index=2 ("length"), length=3 ("index")) -> (w573:T4[])
                  n223 = for {
                    tunnel: w573 -> [w587] mode=indexing
                    tunnel: w576 -> [w586] mode=indexing
                    tunnel: w575 -> [w589] mode=indexing
                    tunnel: w574 -> [w588]
                    tunnel: [w585] -> w567 mode=indexing
                    tunnel: w568 -> [w584]
                    shift-right: [w580] -> w554
                    shift-left: w555 -> [w583]
                    shift-right: [w581] -> w553
                    shift-left: w555 -> [w582]
                    tunnel: w552 -> [w579]
                    n224 = case shown="\"None\"" w589 {
                      selector: w589 -> [_ w625]
                      tunnel: w588 -> [_ w624]
                      tunnel: w587 -> [w593 w610]
                      tunnel: w586 -> [_ w620]
                      tunnel: [w599 w609] -> w585
                      tunnel: w584 -> [_ w622]
                      tunnel: w583 -> [w597 w605]
                      tunnel: w582 -> [w595 w603]
                      tunnel: [w595 w602] -> w581
                      tunnel: [w597 w601] -> w580
                      tunnel: w579 -> [w598 _]
                      frame "None" {
                        n225 = call "IMAQ GetImageSize"("Image"=w598) -> ("Y Resolution"=w594:i32, "X Resolution"=w596:i32)  [unwired: 3 in, 1 out]
                        n226 = Max & Min(x=w597, y=w596) -> (max(x,y)=w591:i32)  [unwired: 1 out]
                        n227 = Max & Min(x=w595, y=w594) -> (max(x,y)=w590:i32)  [unwired: 1 out]
                        n228 = call "IMAQ SetImageSize"("Y Resolution"=w590, "X Resolution"=w591, "Image"=w593) -> ("Image Out"=w592:T4)  [unwired: 2 in, 1 out]
                        n229 = call "IMAQ FillImage"("Pixel Value (U8, U16, I16, Float)"=sgl 0.0, "Image"=w592) -> ("Image Out"=w599:T4)  [unwired: 8 in, 1 out]
                      }
                      frame "Camera 1", Default {
                        w611 = T17 0 items=["Grayscale (U8)", "Grayscale (I16)", "Grayscale (SGL)", "Complex (CSG)", "RGB (U32)", "HSL (U32)", "RGB (U64)", "Grayscale (U16)"] ("Image Type")
                        w621 = T17 2 items=["Grayscale (U8)", "Grayscale (I16)", "Grayscale (SGL)", "Complex (CSG)", "RGB (U32)", "HSL (U32)", "RGB (U64)", "Grayscale (U16)"] ("Image Type")
                        n230 = Decrement(x=w625) -> (x-1=w623:T21)
                        n231 = Index Array(array=w624, index=w623) -> (element=w608:T4)
                        n232 = call "IMAQ GetImageSize"("Image"=w608) -> ("Y Resolution"=w604:i32, "X Resolution"=w606:i32, "error out"=w607:errorcluster)  [unwired: 3 in]
                        n233 = Index Array(array=w620, index #1=0 ("index"), index #2=1 ("index")) -> (element #1=w617:dbl, element #2=w613:dbl)
                        n234 = call "IMAQ Cast Image"("Image Type"=w621, "error in (no error)"=w607, "Image Dst"=w622, "Image Src"=w608) -> ("Image Dst Out"=w616:T4)  [unwired: 6 in, 1 out]
                        n235 = Max & Min(x=w605, y=w606) -> (max(x,y)=w601:i32)  [unwired: 1 out]
                        n236 = Max & Min(x=w603, y=w604) -> (max(x,y)=w602:i32)  [unwired: 1 out]
                        n237 = call "IMAQ Add"("Image Src A"=w616, "Constant"=w617, "Image Dst"=w616) -> ("Image Dst Out"=w614:T4, "error out"=w615:errorcluster)  [unwired: 4 in]
                        n238 = call "IMAQ Multiply"("Image Src A"=w614, "Constant"=w613, "Image Dst"=w614, "error in (no error)"=w615) -> ("Image Dst Out"=w612:T4)  [unwired: 3 in, 1 out]
                        n239 = call "IMAQ Cast Image"("Image Type"=w611, "Image Dst"=w610, "Image Src"=w612) -> ("Image Dst Out"=w609:T4)  [unwired: 7 in, 1 out]
                      }
                    }
                  }
                  n240 = Index Array(array=w567, index #1=0 ("index"), index #2=1 ("index"), index #3=2 ("index")) -> (element #1=w559:T4, element #2=w563:T4, element #3=w562:T4)
                  n241 = call "IMAQ SetImageSize"("Y Resolution"=w553, "X Resolution"=w554, "Image"=w552) -> ("Image Out"=w560:T4)  [unwired: 2 in, 1 out]
                  n242 = call "IMAQ ReplaceColorPlane"("Image Src"=w560, "Color Mode"=w561, "Image Dst"=w560, "Red or Hue Plane"=w559, "Green or Sat Plane"=w563, "Blue or Luma or Val or Inten Plane"=w562) -> ("Image Dst Out"=w558:T4)  [unwired: 8 in, 1 out]
                  n243 = call "IMAQ Copy"("Image Dst"=w556, "Image Src"=w558) -> ("Image Dst Out"=w557:T4)  [unwired: 4 in, 1 out]
                  n244 = property class="ImageControl"(reference=w570, "Value"=w557) -> ()  [unwired: 1 in, 2 out]
                }
              }
            }
          }
          n245 = To Variant(anything=w441) -> (Variant=w440:variant)
        }
        frame 2, Default {
          n246 = stacked-sequence {
            seq-local: [w665 _ _ _] -> [_ _ w777 w1721]
            seq-local: [w664 _ _ _] -> [_ _ w776 w1720]
            seq-local: [w644 _ _ _] -> [_ _ w775 w1719]
            seq-local: [w663 _ _ _] -> [_ _ w774 w1718]
            seq-local: [w662 _ _ _] -> [_ _ w773 w1715]
            seq-local: [w655 _ _ _] -> [_ _ w756 w1717]
            seq-local: [w649 _ _ _] -> [_ _ w751 _]
            seq-local: [_ w725 _ _] -> [_ _ w744 _]
            tunnel: w643 -> [w667 _ w772 w1716]
            tunnel: w642 -> [_ _ w757 _]
            tunnel: w641 -> [w650 w732 w779 w1722]
            tunnel: w640 -> [w651 _ _ _]
            tunnel: w639 -> [_ _ w761 _]
            tunnel: w638 -> [_ _ w771 _]
            tunnel: w637 -> [_ w731 _ _]
            tunnel: w636 -> [_ _ w758 _]
            tunnel: w635 -> [_ _ w770 _]
            tunnel: w634 -> [w654 _ w760 _]
            tunnel: w633 -> [_ _ w755 _]
            tunnel: [w653 _ _ _] -> w632
            tunnel: w631 -> [_ _ w750 _]
            tunnel: w630 -> [_ _ w749 _]
            tunnel: w629 -> [_ _ w748 _]
            tunnel: w628 -> [_ _ w747 _]
            tunnel: w627 -> [_ _ w746 _]
            tunnel: w626 -> [_ _ w745 _]
            frame #0 {
              # "Start acquisition"
              n247 = Index Array(array=w650, index=0) -> (element=w658:T3)
              n248 = for {
                tunnel: w651 -> [w671] mode=indexing
                tunnel: [w669] -> w649 mode=indexing
                tunnel: w650 -> [w670] mode=indexing
                n249 = Unregister For Events(event registration refnum=w671) -> ()  [unwired: 1 in, 1 out]
                n250 = register-events(w670, u32 1 ("BufferInterval")) -> (reference out=w669:refnum<event-registration>)  [unwired: 2 in, 1 out]
              }
              n251 = property class="IMAQdx"(reference=w658, "ActiveAttribute"="CameraAttributes::ImageFormatControl::Width") -> ("ValueU32"=w660:u32)  [unwired: 1 in, 2 out]
              n252 = property class="IMAQdx"(reference=w658, "ActiveAttribute"="CameraAttributes::ImageFormatControl::Height") -> ("ValueU32"=w656:u32)  [unwired: 1 in, 2 out]
              n253 = Not A Number/Path/Refnum?(number/path/refnum=w667) -> (NaN/Path/Refnum?=w666:bool)
              n254 = case shown="False" w666 {
                tunnel: w667 -> [w680 _]
                tunnel: w660 -> [w679 _]
                tunnel: w656 -> [w678 _]
                tunnel: [w677 T11 {"File refnum"=refnum, "Image File Directory"={[], []}, "Big endian?"=FALSE, "IFD Offset Size"=0} ("File data")] -> w645
                tunnel: [w676 refnum<data-value> refnum ("Image data reference")] -> w663
                tunnel: [w675 refnum<queue> refnum ("queue out")] -> w662
                tunnel: [w674 refnum<file> refnum ("refnum out")] -> w664
                tunnel: [w673 "None" ("lowercase file extension")] -> w665
                tunnel: [w672 refnum<queue> refnum ("queue out")] -> w655
                frame False {
                  n255 = call <vilib>:"Get File Extension.vi"("file"=w680) -> ("lowercase file extension"=w673:string)  [unwired: 6 in, 4 out]
                  n256 = case shown="\"'tiff'\", \"tif\"" w673 {
                    tunnel: w680 -> [w700 w712 _]
                    tunnel: w679 -> [w698 _ _]
                    tunnel: w678 -> [w697 _ _]
                    tunnel: [w695 T11 {"File refnum"=refnum, "Image File Directory"={[], []}, "Big endian?"=FALSE, "IFD Offset Size"=0} ("File data") T11 {"File refnum"=refnum, "Image File Directory"={[], []}, "Big endian?"=FALSE, "IFD Offset Size"=0} ("File data")] -> w677
                    tunnel: [w694 refnum<data-value> refnum ("Image data reference") refnum<data-value> refnum ("Image data reference")] -> w676
                    tunnel: [w687 refnum<queue> refnum ("queue out") refnum<queue> refnum ("queue out")] -> w675
                    tunnel: [refnum<file> refnum ("refnum out") w710 refnum<file> refnum ("refnum out")] -> w674
                    tunnel: [w684 w701 refnum<queue> refnum ("queue out")] -> w672
                    frame "'tiff'", "tif" {
                      # "Hack to deal with poor stripe handling"
                      n257 = call "TIFFStream Open.vi"("Bytes per strip"=u32 128000000, "File path"=w700, "Height Pixels"=w697, "Width Pixels"=w698, "Big endian?"=FALSE) -> ("Current and next IFD offset"=w689:u32[], "Image data reference"=w694:refnum<data-value>, "File data"=w695:T11)  [unwired: 3 in, 1 out]
                      n258 = Obtain Queue(max queue size (-1, unlimited)=1, name (unnamed)="TIFF position", element data type=w689) -> (queue out=w688:refnum<queue>, error out=w690:errorcluster)  [unwired: 2 in, 1 out]
                      n259 = Lossy Enqueue Element(queue=w688, element=w689, error in (no error)=w690) -> (queue out=w687:refnum<queue>)  [unwired: 3 out]
                      n260 = Bundle("Camera identity"=enum16{"Camera 1", "Camera 2", "Camera 3"}."Camera 1", "Timestamp"=u64 0) -> (w681:T22)  [unwired: 1 in]
                      n261 = Obtain Queue(max queue size (-1, unlimited)=-1, name (unnamed)="PG Frame order", element data type=w681) -> (queue out=w684:refnum<queue>)  [unwired: 2 in, 2 out]
                    }
                    frame "dat", "u16" {
                      n262 = Bundle("Camera identity"=enum16{"Camera 1", "Camera 2", "Camera 3"}."Camera 1", "Timestamp"=u64 0) -> (w702:T22)  [unwired: 1 in]
                      n263 = Open/Create/Replace File(file path (use dialog)=w712, operation (0:open)=T10."replace or create") -> (refnum out=w710:refnum<file>)  [unwired: 4 in, 2 out]
                      n264 = Obtain Queue(max queue size (-1, unlimited)=-1, name (unnamed)="PG Frame order", element data type=w702) -> (queue out=w701:refnum<queue>)  [unwired: 2 in, 2 out]
                    }
                    frame "None", Default {
                    }
                  }
                }
                frame True {
                }
              }
              n265 = Bundle By Name(cluster=w654, "Camera event refnums"=w649) -> (w652:T6)
              n266 = To Variant(anything=w652) -> (Variant=w653:variant)
              n267 = Obtain Queue(max queue size (-1, unlimited)=1, name (unnamed)="PG TIFF File Data", element data type=w645) -> (queue out=w646:refnum<queue>)  [unwired: 2 in, 2 out]
              n268 = Lossy Enqueue Element(queue=w646, element=w645) -> (queue out=w644:refnum<queue>)  [unwired: 1 in, 3 out]
            }
            frame #1 {
              n269 = for {
                tunnel: w732 -> [w734] mode=indexing
                tunnel: [w733] -> w728 mode=indexing
                n270 = property class="IMAQdx"(reference=w734, "ActiveAttribute"="CameraAttributes::AcquisitionControl::AcquisitionFrameRate") -> ("ValueDBL"=w733:dbl)  [unwired: 1 in, 2 out]
              }
              n271 = for {
                tunnel: w732 -> [w736] mode=indexing
                n272 = disable-structure shown="Enabled" {
                  disable-tunnel: w736 -> [w738 w743]
                  frame Disabled {
                    n273 = property class="IMAQdx"(reference=w738, "ActiveAttribute"="CameraAttributes::AcquisitionControl::TriggerSoftware") -> ()  [unwired: 1 in, 2 out]
                  }
                  frame Enabled {
                    n274 = call <vilib>:"IMAQdx Configure Acquisition.vi"("Number of Buffers"=u32 5, "Continuous?"=IMAQdx_Acquisition_Mode."Continuous", "Session In"=w743) -> ("error out"=w739:errorcluster, "Session Out"=w742:T3)  [unwired: 7 in]
                    n275 = call <vilib>:"IMAQdx Start Acquisition.vi"("error in"=w739, "Session In"=w742) -> ()  [unwired: 8 in, 2 out]
                  }
                }
              }
              n276 = Array Max & Min(array=w728) -> (max value=w730:dbl)  [unwired: 3 out]
              n277 = To Double Precision Float(number=w731) -> (double precision float=w724:dbl)
              n278 = Divide(x=w724, y=w730) -> (x/y=w729:dbl)
              n279 = Multiply(x=w729, y=w728) -> (x*y=w727:dbl[])
              n280 = Round Toward +Infinity(x=w727) -> (ceil(x): smallest int >= x=w726:dbl[])
              n281 = To Unsigned Long Integer(number=w726) -> (unsigned 32bit integer=w725:u32[])
            }
            frame #2 {
              n282 = Obtain Notifier(name (unnamed)="PG Colour", notification data type=FALSE) -> (notifier out=w767:refnum<notifier>, error out=w762:errorcluster)  [unwired: 2 in, 1 out]
              n283 = In Range and Coerce(upper limit=u32 4294967295, x=w744, lower limit=u32 0) -> (coerced(x)=w754:u32[])  [unwired: 1 out]
              n284 = Send Notification(notification=FALSE, notifier=w767, error in (no error)=w762) -> (notifier out=w764:refnum<notifier>)  [unwired: 1 out]
              n285 = To Long Integer(number=w754) -> (32bit integer=w778:i32[])
              n286 = stacked-sequence {
                tunnel: w751 -> [w926 _]
                tunnel: w779 -> [w914 _]
                tunnel: w761 -> [w913 _]
                tunnel: w778 -> [w890 _]
                tunnel: w777 -> [w891 _]
                tunnel: w776 -> [w892 _]
                tunnel: w775 -> [w893 _]
                tunnel: w774 -> [w894 _]
                tunnel: w773 -> [w888 _]
                tunnel: w772 -> [w885 _]
                tunnel: w771 -> [w881 _]
                tunnel: w757 -> [w880 _]
                tunnel: w758 -> [w879 _]
                tunnel: w770 -> [w878 _]
                tunnel: w764 -> [_ w1714]
                tunnel: w756 -> [w895 _]
                tunnel: w755 -> [w907 _]
                tunnel: w750 -> [w876 _]
                tunnel: w749 -> [w882 _]
                tunnel: w748 -> [w905 _]
                tunnel: w747 -> [w902 _]
                tunnel: w745 -> [w884 _]
                frame #0 {
                  n287 = Array Subset(array=w905, index=5, length=3 ("index")) -> (w877:T4[])
                  n288 = Index Array(array=w926, index #1=0 ("index"), index #2=1 ("index"), index #3=2 ("index")) -> (element #1=w911:refnum<event-registration>, element #2=w897:refnum<event-registration>, element #3=w883:refnum<event-registration>)
                  n289 = Index Array(array=w890, index #1=0 ("index"), index #2=1 ("index"), index #3=2 ("index")) -> (element #1=w872:i32, element #2=w871:i32, element #3=w870:i32)
                  n290 = Index Array(array=w907, index #1=0 ("index"), index #2=1 ("index"), index #3=2 ("index")) -> (element #1=w906:T23, element #2=w900:T23, element #3=w889:T23)
                  n291 = Index Array(array=w913, index #1=0 ("index"), index #2=1 ("index"), index #3=2 ("index")) -> (element #1=w919:T4, element #2=w899:T4, element #3=w887:T4)
                  n292 = Index Array(array=w914, index #1=0 ("index"), index #2=1 ("index"), index #3=2 ("index")) -> (element #1=w915:T3, element #2=w898:T3, element #3=w886:T3)
                  n293 = Not A Number/Path/Refnum?(number/path/refnum=w911) -> (NaN/Path/Refnum?=w912:bool)
                  n294 = Not A Number/Path/Refnum?(number/path/refnum=w897) -> (NaN/Path/Refnum?=w901:bool)
                  n295 = Not A Number/Path/Refnum?(number/path/refnum=w883) -> (NaN/Path/Refnum?=w896:bool)
                  n296 = case shown="False" w901 {
                    tunnel: w897 -> [w1209 _]
                    tunnel: w899 -> [w1208 _]
                    tunnel: w898 -> [w1207 _]
                    tunnel: w871 -> [w1206 _]
                    tunnel: w891 -> [w1205 _]
                    tunnel: w892 -> [w1204 _]
                    tunnel: w893 -> [w1203 _]
                    tunnel: w894 -> [w1202 _]
                    tunnel: w888 -> [w1201 _]
                    tunnel: w885 -> [w1200 _]
                    tunnel: w881 -> [w1199 _]
                    tunnel: w880 -> [w1198 _]
                    tunnel: w879 -> [w1197 _]
                    tunnel: w878 -> [w1196 _]
                    tunnel: w895 -> [w1195 _]
                    tunnel: w900 -> [w1194 _]
                    tunnel: w876 -> [w1193 _]
                    tunnel: w882 -> [w1192 _]
                    tunnel: w877 -> [w1191 _]
                    tunnel: w884 -> [w1189 _]
                    frame False {
                      n297 = for {
                        N: w1206 -> [_]
                        tunnel: w1200 -> [w1230]
                        tunnel: w1198 -> [w1229]
                        tunnel: w1209 -> [w1228]
                        tunnel: w1207 -> [w1227]
                        tunnel: w1208 -> [w1226]
                        tunnel: w1199 -> [w1225]
                        tunnel: w1204 -> [w1223]
                        tunnel: w1205 -> [w1222]
                        tunnel: w1203 -> [w1221]
                        tunnel: w1202 -> [w1220]
                        tunnel: w1197 -> [w1219]
                        tunnel: w1201 -> [w1218]
                        tunnel: w1196 -> [w1217]
                        tunnel: w1195 -> [w1216]
                        tunnel: w1194 -> [w1215]
                        tunnel: w1193 -> [w1214]
                        border: u32 0 ("millisecond timer value") -> [_]
                        tunnel: w1192 -> [w1212]
                        tunnel: w1191 -> [w1211]
                        tunnel: w1189 -> [w1210]
                        stop <- w1213 stop-if-true
                        n298 = event shown="[1] <Session Out>: Frame Done" {
                          selector: w1228 -> [_ _]
                          dyn-events: _ -> [_ _]
                          timeout: 1000 -> [_ _]
                          tunnel: w1230 -> [_ _]
                          tunnel: w1229 -> [_ w1264]
                          tunnel: w1227 -> [_ w1258]
                          tunnel: w1226 -> [_ w1254]
                          tunnel: w1225 -> [_ w1257]
                          tunnel: w1223 -> [_ w1262]
                          tunnel: w1222 -> [_ w1234]
                          tunnel: w1221 -> [_ w1261]
                          tunnel: w1220 -> [_ w1260]
                          tunnel: w1219 -> [_ w1259]
                          tunnel: w1218 -> [_ w1255]
                          tunnel: w1217 -> [_ w1251]
                          tunnel: w1216 -> [_ w1256]
                          tunnel: w1215 -> [_ w1239]
                          tunnel: w1214 -> [w1233 w1250]
                          tunnel: [w1231 w1252] -> w1213
                          tunnel: w1212 -> [_ w1237]
                          tunnel: w1211 -> [_ w1236]
                          tunnel: w1210 -> [_ w1235]
                          event Timeout {
                            n299 = event-data() -> ()  [unwired: 1 in, 3 out]
                            n300 = property class="Bool (strict)"(reference=w1233) -> ("Value"=w1232:bool)  [unwired: 1 in, 2 out]
                            n301 = Not(x=w1232) -> (.not. x?=w1231:bool)
                          }
                          event event #0x0 {
                            # "Read data"
                            n302 = event-data() -> ()  [unwired: 1 in, 1 out]
                            n303 = Tick Count (ms)() -> (millisecond timer value=w1238:u32)
                            n304 = feedback #2() -> (w1247:u32)
                            n305 = call "Elapsed time.vi"("Start time (ms)"=w1247, "Current time (ms)"=w1238) -> ("Elapsed time"=w1249:u32)
                            n306 = Greater?(x=w1249, y=w1235) -> (0:w1243:bool)
                            n307 = Select(t=w1238, s=w1243, f=w1247) -> (s? t:f=w1248:u32)
                            n308 = feedback-in #2(w1248) -> ()
                            n309 = call <vilib>:"IMAQdx Get Image2.vi"("Buffer Number Mode (Next)"=IMAQdx_Buffer_Number_Mode."Last New", "Image In"=w1254, "Session In"=w1258) -> ("error out"=w1241:errorcluster, "Image Out"=w1242:T4)  [unwired: 5 in, 2 out]
                            n310 = Not A Number/Path/Refnum?(number/path/refnum=w1264) -> (NaN/Path/Refnum?=w1245:bool)
                            n311 = Not(x=w1243) -> (.not. x?=w1244:bool)
                            n312 = Or(x=w1245, y=w1244) -> (x .or. y?=w1246:bool)
                            n313 = case shown="\"dat\", \"u16\"" w1234 {
                              tunnel: w1242 -> [w1266 w1310 w1313]
                              tunnel: w1262 -> [_ _ w1314]
                              tunnel: w1261 -> [w1267 _ _]
                              tunnel: w1260 -> [w1268 _ _]
                              tunnel: w1255 -> [w1272 _ _]
                              tunnel: w1251 -> [w1271 _ w1318]
                              tunnel: w1256 -> [w1270 _ w1315]
                              tunnel: w1241 -> [w1269 _ w1317]
                              tunnel: [w1265 w1310 w1313] -> w1240
                              frame "'tiff'", "tif" {
                                n314 = stacked-sequence {
                                tunnel: w1272 -> [_ w1286 _ _]
                                tunnel: w1271 -> [w1273 _ _ w1303]
                                tunnel: w1270 -> [_ _ w1301 _]
                                tunnel: w1269 -> [_ w1281 _ _]
                                tunnel: w1268 -> [_ w1280 _ _]
                                tunnel: w1267 -> [_ w1276 _ _]
                                tunnel: w1266 -> [_ w1278 w1292 _]
                                tunnel: [_ w1278 _ _] -> w1265
                                frame #0 {
                                n315 = call <vilib>:"Acquire Semaphore.vi"("semaphore"=w1273) -> ()  [unwired: 4 in, 3 out]
                                }
                                frame #1 {
                                n316 = Preview Queue Element(queue=w1276) -> (queue out=w1277:refnum<queue>, element=w1275:T11)  [unwired: 2 in, 2 out]
                                n317 = in-place {
                                in-place-border: w1278 -> [w1289]
                                in-place-border: w1281 -> [w1288]
                                n318 = in-place-dvr #3(w1280) -> ()  [unwired: 2 out]
                                n319 = call "IMAQ ImageToArray"("error in (no error)"=w1288, "Image"=w1289) -> ("Image Pixels (I16)"=w1287:i16[][])  [unwired: 2 in, 4 out]
                                n320 = in-place-dvr #3(w1287) -> (w1279:refnum<data-value>)  [unwired: 1 out]
                                }
                                n321 = Preview Queue Element(queue=w1286) -> (queue out=w1284:refnum<queue>, element=w1285:u32[])  [unwired: 2 in, 2 out]
                                n322 = call "TIFFStream Write.vi"("File data"=w1275, "Last image in file?"=FALSE, "Current and next IFD offset in"=w1285, "Image data reference"=w1279) -> ("Current and next IFD offset out"=w1283:u32[], "File data out"=w1274:T11)  [unwired: 5 in, 1 out]
                                n323 = Lossy Enqueue Element(queue=w1277, element=w1274) -> ()  [unwired: 1 in, 4 out]
                                n324 = Lossy Enqueue Element(queue=w1284, element=w1283) -> ()  [unwired: 1 in, 4 out]
                                }
                                frame #2 {
                                w1295 = u32 0
                                n325 = call "IMAQ Read Custom Data"("Key"="IMAQdxReceiveTimestampHigh", "Image"=w1292) -> ("Custom Data Out"=w1299:string, "Image (duplicate)"=w1298:T4)  [unwired: 7 in, 1 out]
                                n326 = Unflatten From String(type=w1295, binary string=w1299) -> (value=w1294:u32)  [unwired: 3 in, 2 out]
                                n327 = call "IMAQ Read Custom Data"("Key"="IMAQdxReceiveTimestampLow", "Image"=w1298) -> ("Custom Data Out"=w1296:string)  [unwired: 7 in, 2 out]
                                n328 = Unflatten From String(type=w1295, binary string=w1296) -> (value=w1293:u32)  [unwired: 3 in, 2 out]
                                n329 = Join Numbers(hi=w1294, lo=w1293) -> ((hi.lo)=w1290:u64)
                                n330 = Bundle("element"=enum16{"Camera 1", "Camera 2", "Camera 3"}."Camera 2", w1290) -> (w1291:T24)  [unwired: 1 in]
                                n331 = Enqueue Element(queue=w1301, element=w1291) -> ()  [unwired: 2 in, 3 out]
                                }
                                frame #3 {
                                n332 = call <vilib>:"Release Semaphore.vi"("semaphore"=w1303) -> ()  [unwired: 5 in, 2 out]
                                }
                                }
                              }
                              frame "None", Default {
                                w1306 = u32 0
                                n333 = call "IMAQ Read Custom Data"("Key"="IMAQdxReceiveTimestampHigh", "Image"=w1310) -> ("Custom Data Out"=w1311:string, "Image (duplicate)"=w1309:T4)  [unwired: 7 in, 1 out]
                                n334 = Unflatten From String(type=w1306, binary string=w1311) -> (value=w1305:u32)  [unwired: 3 in, 2 out]
                                n335 = call "IMAQ Read Custom Data"("Key"="IMAQdxReceiveTimestampLow", "Image"=w1309) -> ("Custom Data Out"=w1307:string)  [unwired: 7 in, 2 out]
                                n336 = Unflatten From String(type=w1306, binary string=w1307) -> (value=w1304:u32)  [unwired: 3 in, 2 out]
                                n337 = Join Numbers(hi=w1305, lo=w1304) -> ()  [unwired: 1 out]
                              }
                              frame "dat", "u16" {
                                n338 = call "IMAQ ImageToArray"("error in (no error)"=w1317, "Image"=w1313) -> ("Image Pixels (I16)"=w1316:i16[][])  [unwired: 2 in, 4 out]
                                n339 = stacked-sequence {
                                seq-local: [_ _ w1323 _ _] -> [_ _ _ w1333 _]
                                tunnel: w1316 -> [_ w1321 _ _ _]
                                tunnel: w1314 -> [_ w1320 _ _ _]
                                tunnel: w1318 -> [w1319 _ _ _ w1337]
                                tunnel: w1315 -> [_ _ _ w1336 _]
                                tunnel: w1313 -> [_ _ w1324 _ _]
                                frame #0 {
                                n340 = call <vilib>:"Acquire Semaphore.vi"("semaphore"=w1319) -> ()  [unwired: 4 in, 3 out]
                                }
                                frame #1 {
                                n341 = Write to Binary File(file (use dialog)=w1320, data=w1321, 5:FALSE ("prepend array or string size? (T)")) -> ()  [unwired: 3 in, 3 out]
                                }
                                frame #2 {
                                w1327 = u32 0
                                n342 = call "IMAQ Read Custom Data"("Key"="IMAQdxReceiveTimestampHigh", "Image"=w1324) -> ("Custom Data Out"=w1331:string, "Image (duplicate)"=w1330:T4)  [unwired: 7 in, 1 out]
                                n343 = Unflatten From String(type=w1327, binary string=w1331) -> (value=w1326:u32)  [unwired: 3 in, 2 out]
                                n344 = call "IMAQ Read Custom Data"("Key"="IMAQdxReceiveTimestampLow", "Image"=w1330) -> ("Custom Data Out"=w1328:string)  [unwired: 7 in, 2 out]
                                n345 = Unflatten From String(type=w1327, binary string=w1328) -> (value=w1325:u32)  [unwired: 3 in, 2 out]
                                n346 = Join Numbers(hi=w1326, lo=w1325) -> ((hi.lo)=w1323:u64)
                                }
                                frame #3 {
                                n347 = Bundle("element"=enum16{"Camera 1", "Camera 2", "Camera 3"}."Camera 2", w1333) -> (w1335:T24)  [unwired: 1 in]
                                n348 = Enqueue Element(queue=w1336, element=w1335) -> ()  [unwired: 2 in, 3 out]
                                }
                                frame #4 {
                                n349 = call <vilib>:"Release Semaphore.vi"("semaphore"=w1337) -> ()  [unwired: 5 in, 2 out]
                                }
                                }
                              }
                            }
                            n350 = case shown="False" w1246 {
                              tunnel: w1264 -> [w1343 _]
                              tunnel: w1257 -> [w1344 _]
                              tunnel: w1259 -> [w1342 _]
                              tunnel: w1240 -> [w1341 _]
                              tunnel: w1239 -> [w1338 _]
                              tunnel: w1237 -> [w1340 _]
                              tunnel: w1236 -> [w1339 _]
                              frame False {
                                n351 = case shown="2" w1344 {
                                tunnel: w1343 -> [_ _ w1405]
                                tunnel: w1342 -> [_ _ w1404]
                                tunnel: w1341 -> [_ w1348 w1401]
                                tunnel: w1340 -> [_ w1347 _]
                                tunnel: w1339 -> [_ w1346 _]
                                tunnel: w1338 -> [_ w1345 w1400]
                                frame -1, Default {
                                }
                                frame 0 {
                                n352 = case shown="\"Anticlockwise, Flip UD\"" w1345 {
                                tunnel: w1348 -> [w1355 w1358 w1361 w1364 w1371 w1378 w1381 w1390 w1397]
                                tunnel: [w1355 w1357 w1360 w1362 w1367 w1374 w1382 w1386 w1393] -> w1349
                                frame "No rotation, No flip", Default {
                                }
                                frame "No rotation, Flip UD" {
                                w1356 = u32 0 items=["Horizontal", "Vertical", "Central", "1st Diagonal", "2nd Diagonal"] ("Type of Symmetry")
                                n353 = call "IMAQ Symmetry"("Type of Symmetry"=w1356, "Image Dst"=w1358, "Image Src"=w1358) -> ("Image Dst Out"=w1357:T4)  [unwired: 2 in, 1 out]
                                }
                                frame "No rotation, Flip LR" {
                                w1359 = u32 1 items=["Horizontal", "Vertical", "Central", "1st Diagonal", "2nd Diagonal"] ("Type of Symmetry")
                                n354 = call "IMAQ Symmetry"("Type of Symmetry"=w1359, "Image Dst"=w1361, "Image Src"=w1361) -> ("Image Dst Out"=w1360:T4)  [unwired: 2 in, 1 out]
                                }
                                frame "Clockwise, No flip" {
                                n355 = call "IMAQ Rotate"("Use Bilinear Interpolation"=FALSE, "Maintain Size"=FALSE, "Angle (degrees)"=sgl 270.0, "Image Dst"=w1364, "Image Src"=w1364) -> ("Image Dst Out"=w1362:T4)  [unwired: 5 in, 1 out]
                                }
                                frame "Clockwise, Flip UD" {
                                w1369 = u32 0 items=["Horizontal", "Vertical", "Central", "1st Diagonal", "2nd Diagonal"] ("Type of Symmetry")
                                n356 = call "IMAQ Rotate"("Use Bilinear Interpolation"=FALSE, "Maintain Size"=FALSE, "Angle (degrees)"=sgl 270.0, "Image Dst"=w1371, "Image Src"=w1371) -> ("Image Dst Out"=w1368:T4)  [unwired: 5 in, 1 out]
                                n357 = call "IMAQ Symmetry"("Type of Symmetry"=w1369, "Image Dst"=w1368, "Image Src"=w1368) -> ("Image Dst Out"=w1367:T4)  [unwired: 2 in, 1 out]
                                }
                                frame "Clockwise, Flip LR" {
                                w1376 = u32 1 items=["Horizontal", "Vertical", "Central", "1st Diagonal", "2nd Diagonal"] ("Type of Symmetry")
                                n358 = call "IMAQ Rotate"("Use Bilinear Interpolation"=FALSE, "Maintain Size"=FALSE, "Angle (degrees)"=sgl 270.0, "Image Dst"=w1378, "Image Src"=w1378) -> ("Image Dst Out"=w1375:T4)  [unwired: 5 in, 1 out]
                                n359 = call "IMAQ Symmetry"("Type of Symmetry"=w1376, "Image Dst"=w1375, "Image Src"=w1375) -> ("Image Dst Out"=w1374:T4)  [unwired: 2 in, 1 out]
                                }
                                frame "Anticlockwise, No flip" {
                                n360 = call "IMAQ Rotate"("Use Bilinear Interpolation"=FALSE, "Maintain Size"=FALSE, "Angle (degrees)"=sgl 90.0, "Image Dst"=w1381, "Image Src"=w1381) -> ("Image Dst Out"=w1382:T4)  [unwired: 5 in, 1 out]
                                }
                                frame "Anticlockwise, Flip UD" {
                                w1388 = u32 0 items=["Horizontal", "Vertical", "Central", "1st Diagonal", "2nd Diagonal"] ("Type of Symmetry")
                                n361 = call "IMAQ Rotate"("Use Bilinear Interpolation"=FALSE, "Maintain Size"=FALSE, "Angle (degrees)"=sgl 90.0, "Image Dst"=w1390, "Image Src"=w1390) -> ("Image Dst Out"=w1387:T4)  [unwired: 5 in, 1 out]
                                n362 = call "IMAQ Symmetry"("Type of Symmetry"=w1388, "Image Dst"=w1387, "Image Src"=w1387) -> ("Image Dst Out"=w1386:T4)  [unwired: 2 in, 1 out]
                                }
                                frame "Anticlockwise, Flip LR" {
                                w1395 = u32 1 items=["Horizontal", "Vertical", "Central", "1st Diagonal", "2nd Diagonal"] ("Type of Symmetry")
                                n363 = call "IMAQ Rotate"("Use Bilinear Interpolation"=FALSE, "Maintain Size"=FALSE, "Angle (degrees)"=sgl 90.0, "Image Dst"=w1397, "Image Src"=w1397) -> ("Image Dst Out"=w1394:T4)  [unwired: 5 in, 1 out]
                                n364 = call "IMAQ Symmetry"("Type of Symmetry"=w1395, "Image Dst"=w1394, "Image Src"=w1394) -> ("Image Dst Out"=w1393:T4)  [unwired: 2 in, 1 out]
                                }
                                }
                                n365 = for {
                                tunnel: w1349 -> [w1352]
                                tunnel: w1347 -> [w1351] mode=indexing
                                tunnel: w1346 -> [w1350] mode=indexing
                                n366 = case shown="\"Camera 2\"" w1351 {
                                tunnel: w1352 -> [_ w1354]
                                tunnel: w1350 -> [_ w1353]
                                frame "None", Default {
                                }
                                frame "Camera 2" {
                                n367 = call "IMAQ Copy"("Image Dst"=w1353, "Image Src"=w1354) -> ()  [unwired: 4 in, 2 out]
                                }
                                }
                                }
                                }
                                frame 2 {
                                n368 = case shown="\"Anticlockwise, Flip UD\"" w1400 {
                                tunnel: w1401 -> [w1406 w1409 w1412 w1415 w1422 w1429 w1432 w1441 w1448]
                                tunnel: [w1406 w1408 w1411 w1413 w1418 w1425 w1433 w1437 w1444] -> w1402
                                frame "No rotation, No flip", Default {
                                }
                                frame "No rotation, Flip UD" {
                                w1407 = u32 0 items=["Horizontal", "Vertical", "Central", "1st Diagonal", "2nd Diagonal"] ("Type of Symmetry")
                                n369 = call "IMAQ Symmetry"("Type of Symmetry"=w1407, "Image Dst"=w1409, "Image Src"=w1409) -> ("Image Dst Out"=w1408:T4)  [unwired: 2 in, 1 out]
                                }
                                frame "No rotation, Flip LR" {
                                w1410 = u32 1 items=["Horizontal", "Vertical", "Central", "1st Diagonal", "2nd Diagonal"] ("Type of Symmetry")
                                n370 = call "IMAQ Symmetry"("Type of Symmetry"=w1410, "Image Dst"=w1412, "Image Src"=w1412) -> ("Image Dst Out"=w1411:T4)  [unwired: 2 in, 1 out]
                                }
                                frame "Clockwise, No flip" {
                                n371 = call "IMAQ Rotate"("Use Bilinear Interpolation"=FALSE, "Maintain Size"=FALSE, "Angle (degrees)"=sgl 270.0, "Image Dst"=w1415, "Image Src"=w1415) -> ("Image Dst Out"=w1413:T4)  [unwired: 5 in, 1 out]
                                }
                                frame "Clockwise, Flip UD" {
                                w1420 = u32 0 items=["Horizontal", "Vertical", "Central", "1st Diagonal", "2nd Diagonal"] ("Type of Symmetry")
                                n372 = call "IMAQ Rotate"("Use Bilinear Interpolation"=FALSE, "Maintain Size"=FALSE, "Angle (degrees)"=sgl 270.0, "Image Dst"=w1422, "Image Src"=w1422) -> ("Image Dst Out"=w1419:T4)  [unwired: 5 in, 1 out]
                                n373 = call "IMAQ Symmetry"("Type of Symmetry"=w1420, "Image Dst"=w1419, "Image Src"=w1419) -> ("Image Dst Out"=w1418:T4)  [unwired: 2 in, 1 out]
                                }
                                frame "Clockwise, Flip LR" {
                                w1427 = u32 1 items=["Horizontal", "Vertical", "Central", "1st Diagonal", "2nd Diagonal"] ("Type of Symmetry")
                                n374 = call "IMAQ Rotate"("Use Bilinear Interpolation"=FALSE, "Maintain Size"=FALSE, "Angle (degrees)"=sgl 270.0, "Image Dst"=w1429, "Image Src"=w1429) -> ("Image Dst Out"=w1426:T4)  [unwired: 5 in, 1 out]
                                n375 = call "IMAQ Symmetry"("Type of Symmetry"=w1427, "Image Dst"=w1426, "Image Src"=w1426) -> ("Image Dst Out"=w1425:T4)  [unwired: 2 in, 1 out]
                                }
                                frame "Anticlockwise, No flip" {
                                n376 = call "IMAQ Rotate"("Use Bilinear Interpolation"=FALSE, "Maintain Size"=FALSE, "Angle (degrees)"=sgl 90.0, "Image Dst"=w1432, "Image Src"=w1432) -> ("Image Dst Out"=w1433:T4)  [unwired: 5 in, 1 out]
                                }
                                frame "Anticlockwise, Flip UD" {
                                w1439 = u32 0 items=["Horizontal", "Vertical", "Central", "1st Diagonal", "2nd Diagonal"] ("Type of Symmetry")
                                n377 = call "IMAQ Rotate"("Use Bilinear Interpolation"=FALSE, "Maintain Size"=FALSE, "Angle (degrees)"=sgl 90.0, "Image Dst"=w1441, "Image Src"=w1441) -> ("Image Dst Out"=w1438:T4)  [unwired: 5 in, 1 out]
                                n378 = call "IMAQ Symmetry"("Type of Symmetry"=w1439, "Image Dst"=w1438, "Image Src"=w1438) -> ("Image Dst Out"=w1437:T4)  [unwired: 2 in, 1 out]
                                }
                                frame "Anticlockwise, Flip LR" {
                                w1446 = u32 1 items=["Horizontal", "Vertical", "Central", "1st Diagonal", "2nd Diagonal"] ("Type of Symmetry")
                                n379 = call "IMAQ Rotate"("Use Bilinear Interpolation"=FALSE, "Maintain Size"=FALSE, "Angle (degrees)"=sgl 90.0, "Image Dst"=w1448, "Image Src"=w1448) -> ("Image Dst Out"=w1445:T4)  [unwired: 5 in, 1 out]
                                n380 = call "IMAQ Symmetry"("Type of Symmetry"=w1446, "Image Dst"=w1445, "Image Src"=w1445) -> ("Image Dst Out"=w1444:T4)  [unwired: 2 in, 1 out]
                                }
                                }
                                n381 = call "IMAQ Copy"("Image Dst"=w1405, "Image Src"=w1402) -> ("Image Dst Out"=w1403:T4)  [unwired: 4 in, 1 out]
                                n382 = property class="ImageControl"(reference=w1404, "Value"=w1403) -> ()  [unwired: 1 in, 2 out]
                                }
                                }
                              }
                              frame True {
                              }
                            }
                            n383 = property class="Bool (strict)"(reference=w1250) -> ("Value"=w1253:bool)  [unwired: 1 in, 2 out]
                            n384 = Not(x=w1253) -> (.not. x?=w1252:bool)
                          }
                        }
                      }
                    }
                    frame True {
                    }
                  }
                  n385 = case shown="False" w896 {
                    tunnel: w883 -> [w947 _]
                    tunnel: w887 -> [w946 _]
                    tunnel: w886 -> [w945 _]
                    tunnel: w870 -> [w944 _]
                    tunnel: w891 -> [w943 _]
                    tunnel: w892 -> [w942 _]
                    tunnel: w893 -> [w941 _]
                    tunnel: w894 -> [w940 _]
                    tunnel: w888 -> [w939 _]
                    tunnel: w885 -> [w938 _]
                    tunnel: w881 -> [w937 _]
                    tunnel: w880 -> [w936 _]
                    tunnel: w879 -> [w935 _]
                    tunnel: w878 -> [w934 _]
                    tunnel: w895 -> [w933 _]
                    tunnel: w889 -> [w932 _]
                    tunnel: w876 -> [w931 _]
                    tunnel: w882 -> [w930 _]
                    tunnel: w877 -> [w929 _]
                    tunnel: w884 -> [w927 _]
                    frame False {
                      n386 = for {
                        N: w944 -> [_]
                        tunnel: w938 -> [w968]
                        tunnel: w936 -> [w967]
                        tunnel: w947 -> [w966]
                        tunnel: w945 -> [w965]
                        tunnel: w946 -> [w964]
                        tunnel: w937 -> [w963]
                        tunnel: w942 -> [w961]
                        tunnel: w943 -> [w960]
                        tunnel: w941 -> [w959]
                        tunnel: w940 -> [w958]
                        tunnel: w935 -> [w957]
                        tunnel: w939 -> [w956]
                        tunnel: w934 -> [w955]
                        tunnel: w933 -> [w954]
                        tunnel: w932 -> [w953]
                        tunnel: w931 -> [w952]
                        border: u32 0 ("millisecond timer value") -> [_]
                        tunnel: w930 -> [w950]
                        tunnel: w929 -> [w949]
                        tunnel: w927 -> [w948]
                        stop <- w951 stop-if-true
                        n387 = event shown="[1] <Session Out>: Frame Done" {
                          selector: w966 -> [_ _]
                          dyn-events: _ -> [_ _]
                          timeout: 1000 -> [_ _]
                          tunnel: w968 -> [_ _]
                          tunnel: w967 -> [_ w1002]
                          tunnel: w965 -> [_ w996]
                          tunnel: w964 -> [_ w992]
                          tunnel: w963 -> [_ w995]
                          tunnel: w961 -> [_ w1000]
                          tunnel: w960 -> [_ w972]
                          tunnel: w959 -> [_ w999]
                          tunnel: w958 -> [_ w998]
                          tunnel: w957 -> [_ w997]
                          tunnel: w956 -> [_ w993]
                          tunnel: w955 -> [_ w989]
                          tunnel: w954 -> [_ w994]
                          tunnel: w953 -> [_ w977]
                          tunnel: w952 -> [w971 w988]
                          tunnel: [w969 w990] -> w951
                          tunnel: w950 -> [_ w975]
                          tunnel: w949 -> [_ w974]
                          tunnel: w948 -> [_ w973]
                          event Timeout {
                            n388 = event-data() -> ()  [unwired: 1 in, 3 out]
                            n389 = property class="Bool (strict)"(reference=w971) -> ("Value"=w970:bool)  [unwired: 1 in, 2 out]
                            n390 = Not(x=w970) -> (.not. x?=w969:bool)
                          }
                          event event #0x0 {
                            # "Read data"
                            n391 = event-data() -> ()  [unwired: 1 in, 1 out]
                            n392 = Tick Count (ms)() -> (millisecond timer value=w976:u32)
                            n393 = feedback #4() -> (w985:u32)
                            n394 = call "Elapsed time.vi"("Start time (ms)"=w985, "Current time (ms)"=w976) -> ("Elapsed time"=w987:u32)
                            n395 = Greater?(x=w987, y=w973) -> (0:w981:bool)
                            n396 = Select(t=w976, s=w981, f=w985) -> (s? t:f=w986:u32)
                            n397 = feedback-in #4(w986) -> ()
                            n398 = call <vilib>:"IMAQdx Get Image2.vi"("Buffer Number Mode (Next)"=IMAQdx_Buffer_Number_Mode."Last New", "Image In"=w992, "Session In"=w996) -> ("error out"=w979:errorcluster, "Image Out"=w980:T4)  [unwired: 5 in, 2 out]
                            n399 = Not A Number/Path/Refnum?(number/path/refnum=w1002) -> (NaN/Path/Refnum?=w983:bool)
                            n400 = Not(x=w981) -> (.not. x?=w982:bool)
                            n401 = Or(x=w983, y=w982) -> (x .or. y?=w984:bool)
                            n402 = case shown="\"'tiff'\", \"tif\"" w972 {
                              tunnel: w980 -> [w1004 w1048 w1051]
                              tunnel: w1000 -> [_ _ w1052]
                              tunnel: w999 -> [w1005 _ _]
                              tunnel: w998 -> [w1006 _ _]
                              tunnel: w993 -> [w1010 _ _]
                              tunnel: w989 -> [w1009 _ w1056]
                              tunnel: w994 -> [w1008 _ w1053]
                              tunnel: w979 -> [w1007 _ w1055]
                              tunnel: [w1003 w1048 w1051] -> w978
                              frame "'tiff'", "tif" {
                                n403 = stacked-sequence {
                                tunnel: w1010 -> [_ w1024 _ _]
                                tunnel: w1009 -> [w1011 _ _ w1041]
                                tunnel: w1008 -> [_ _ w1039 _]
                                tunnel: w1007 -> [_ w1019 _ _]
                                tunnel: w1006 -> [_ w1018 _ _]
                                tunnel: w1005 -> [_ w1014 _ _]
                                tunnel: w1004 -> [_ w1016 w1030 _]
                                tunnel: [_ w1016 _ _] -> w1003
                                frame #0 {
                                n404 = call <vilib>:"Acquire Semaphore.vi"("semaphore"=w1011) -> ()  [unwired: 4 in, 3 out]
                                }
                                frame #1 {
                                n405 = Preview Queue Element(queue=w1014) -> (queue out=w1015:refnum<queue>, element=w1013:T11)  [unwired: 2 in, 2 out]
                                n406 = in-place {
                                in-place-border: w1016 -> [w1027]
                                in-place-border: w1019 -> [w1026]
                                n407 = in-place-dvr #5(w1018) -> ()  [unwired: 2 out]
                                n408 = call "IMAQ ImageToArray"("error in (no error)"=w1026, "Image"=w1027) -> ("Image Pixels (I16)"=w1025:i16[][])  [unwired: 2 in, 4 out]
                                n409 = in-place-dvr #5(w1025) -> (w1017:refnum<data-value>)  [unwired: 1 out]
                                }
                                n410 = Preview Queue Element(queue=w1024) -> (queue out=w1022:refnum<queue>, element=w1023:u32[])  [unwired: 2 in, 2 out]
                                n411 = call "TIFFStream Write.vi"("File data"=w1013, "Last image in file?"=FALSE, "Current and next IFD offset in"=w1023, "Image data reference"=w1017) -> ("Current and next IFD offset out"=w1021:u32[], "File data out"=w1012:T11)  [unwired: 5 in, 1 out]
                                n412 = Lossy Enqueue Element(queue=w1015, element=w1012) -> ()  [unwired: 1 in, 4 out]
                                n413 = Lossy Enqueue Element(queue=w1022, element=w1021) -> ()  [unwired: 1 in, 4 out]
                                }
                                frame #2 {
                                w1033 = u32 0
                                n414 = call "IMAQ Read Custom Data"("Key"="IMAQdxReceiveTimestampHigh", "Image"=w1030) -> ("Custom Data Out"=w1037:string, "Image (duplicate)"=w1036:T4)  [unwired: 7 in, 1 out]
                                n415 = Unflatten From String(type=w1033, binary string=w1037) -> (value=w1032:u32)  [unwired: 3 in, 2 out]
                                n416 = call "IMAQ Read Custom Data"("Key"="IMAQdxReceiveTimestampLow", "Image"=w1036) -> ("Custom Data Out"=w1034:string)  [unwired: 7 in, 2 out]
                                n417 = Unflatten From String(type=w1033, binary string=w1034) -> (value=w1031:u32)  [unwired: 3 in, 2 out]
                                n418 = Join Numbers(hi=w1032, lo=w1031) -> ((hi.lo)=w1028:u64)
                                n419 = Bundle("element"=enum16{"Camera 1", "Camera 2", "Camera 3"}."Camera 3", w1028) -> (w1029:T24)  [unwired: 1 in]
                                n420 = Enqueue Element(queue=w1039, element=w1029) -> ()  [unwired: 2 in, 3 out]
                                }
                                frame #3 {
                                n421 = call <vilib>:"Release Semaphore.vi"("semaphore"=w1041) -> ()  [unwired: 5 in, 2 out]
                                }
                                }
                              }
                              frame "None", Default {
                                w1044 = u32 0
                                n422 = call "IMAQ Read Custom Data"("Key"="IMAQdxReceiveTimestampHigh", "Image"=w1048) -> ("Custom Data Out"=w1049:string, "Image (duplicate)"=w1047:T4)  [unwired: 7 in, 1 out]
                                n423 = Unflatten From String(type=w1044, binary string=w1049) -> (value=w1043:u32)  [unwired: 3 in, 2 out]
                                n424 = call "IMAQ Read Custom Data"("Key"="IMAQdxReceiveTimestampLow", "Image"=w1047) -> ("Custom Data Out"=w1045:string)  [unwired: 7 in, 2 out]
                                n425 = Unflatten From String(type=w1044, binary string=w1045) -> (value=w1042:u32)  [unwired: 3 in, 2 out]
                                n426 = Join Numbers(hi=w1043, lo=w1042) -> ()  [unwired: 1 out]
                              }
                              frame "dat", "u16" {
                                n427 = call "IMAQ ImageToArray"("error in (no error)"=w1055, "Image"=w1051) -> ("Image Pixels (I16)"=w1054:i16[][])  [unwired: 2 in, 4 out]
                                n428 = stacked-sequence {
                                seq-local: [_ _ w1061 _ _] -> [_ _ _ w1071 _]
                                tunnel: w1054 -> [_ w1059 _ _ _]
                                tunnel: w1052 -> [_ w1058 _ _ _]
                                tunnel: w1056 -> [w1057 _ _ _ w1075]
                                tunnel: w1053 -> [_ _ _ w1074 _]
                                tunnel: w1051 -> [_ _ w1062 _ _]
                                frame #0 {
                                n429 = call <vilib>:"Acquire Semaphore.vi"("semaphore"=w1057) -> ()  [unwired: 4 in, 3 out]
                                }
                                frame #1 {
                                n430 = Write to Binary File(file (use dialog)=w1058, data=w1059, 5:FALSE ("prepend array or string size? (T)")) -> ()  [unwired: 3 in, 3 out]
                                }
                                frame #2 {
                                w1065 = u32 0
                                n431 = call "IMAQ Read Custom Data"("Key"="IMAQdxReceiveTimestampHigh", "Image"=w1062) -> ("Custom Data Out"=w1069:string, "Image (duplicate)"=w1068:T4)  [unwired: 7 in, 1 out]
                                n432 = Unflatten From String(type=w1065, binary string=w1069) -> (value=w1064:u32)  [unwired: 3 in, 2 out]
                                n433 = call "IMAQ Read Custom Data"("Key"="IMAQdxReceiveTimestampLow", "Image"=w1068) -> ("Custom Data Out"=w1066:string)  [unwired: 7 in, 2 out]
                                n434 = Unflatten From String(type=w1065, binary string=w1066) -> (value=w1063:u32)  [unwired: 3 in, 2 out]
                                n435 = Join Numbers(hi=w1064, lo=w1063) -> ((hi.lo)=w1061:u64)
                                }
                                frame #3 {
                                n436 = Bundle("element"=enum16{"Camera 1", "Camera 2", "Camera 3"}."Camera 3", w1071) -> (w1073:T24)  [unwired: 1 in]
                                n437 = Enqueue Element(queue=w1074, element=w1073) -> ()  [unwired: 2 in, 3 out]
                                }
                                frame #4 {
                                n438 = call <vilib>:"Release Semaphore.vi"("semaphore"=w1075) -> ()  [unwired: 5 in, 2 out]
                                }
                                }
                              }
                            }
                            n439 = case shown="False" w984 {
                              tunnel: w1002 -> [w1081 _]
                              tunnel: w995 -> [w1082 _]
                              tunnel: w997 -> [w1080 _]
                              tunnel: w978 -> [w1079 _]
                              tunnel: w977 -> [w1076 _]
                              tunnel: w975 -> [w1078 _]
                              tunnel: w974 -> [w1077 _]
                              frame False {
                                n440 = case shown="0" w1082 {
                                tunnel: w1081 -> [_ _ w1143]
                                tunnel: w1080 -> [_ _ w1142]
                                tunnel: w1079 -> [_ w1086 w1139]
                                tunnel: w1078 -> [_ w1085 _]
                                tunnel: w1077 -> [_ w1084 _]
                                tunnel: w1076 -> [_ w1083 w1138]
                                frame -1, Default {
                                }
                                frame 0 {
                                n441 = case shown="\"Anticlockwise, Flip UD\"" w1083 {
                                tunnel: w1086 -> [w1093 w1096 w1099 w1102 w1109 w1116 w1119 w1128 w1135]
                                tunnel: [w1093 w1095 w1098 w1100 w1105 w1112 w1120 w1124 w1131] -> w1087
                                frame "No rotation, No flip", Default {
                                }
                                frame "No rotation, Flip UD" {
                                w1094 = u32 0 items=["Horizontal", "Vertical", "Central", "1st Diagonal", "2nd Diagonal"] ("Type of Symmetry")
                                n442 = call "IMAQ Symmetry"("Type of Symmetry"=w1094, "Image Dst"=w1096, "Image Src"=w1096) -> ("Image Dst Out"=w1095:T4)  [unwired: 2 in, 1 out]
                                }
                                frame "No rotation, Flip LR" {
                                w1097 = u32 1 items=["Horizontal", "Vertical", "Central", "1st Diagonal", "2nd Diagonal"] ("Type of Symmetry")
                                n443 = call "IMAQ Symmetry"("Type of Symmetry"=w1097, "Image Dst"=w1099, "Image Src"=w1099) -> ("Image Dst Out"=w1098:T4)  [unwired: 2 in, 1 out]
                                }
                                frame "Clockwise, No flip" {
                                n444 = call "IMAQ Rotate"("Use Bilinear Interpolation"=FALSE, "Maintain Size"=FALSE, "Angle (degrees)"=sgl 270.0, "Image Dst"=w1102, "Image Src"=w1102) -> ("Image Dst Out"=w1100:T4)  [unwired: 5 in, 1 out]
                                }
                                frame "Clockwise, Flip UD" {
                                w1107 = u32 0 items=["Horizontal", "Vertical", "Central", "1st Diagonal", "2nd Diagonal"] ("Type of Symmetry")
                                n445 = call "IMAQ Rotate"("Use Bilinear Interpolation"=FALSE, "Maintain Size"=FALSE, "Angle (degrees)"=sgl 270.0, "Image Dst"=w1109, "Image Src"=w1109) -> ("Image Dst Out"=w1106:T4)  [unwired: 5 in, 1 out]
                                n446 = call "IMAQ Symmetry"("Type of Symmetry"=w1107, "Image Dst"=w1106, "Image Src"=w1106) -> ("Image Dst Out"=w1105:T4)  [unwired: 2 in, 1 out]
                                }
                                frame "Clockwise, Flip LR" {
                                w1114 = u32 1 items=["Horizontal", "Vertical", "Central", "1st Diagonal", "2nd Diagonal"] ("Type of Symmetry")
                                n447 = call "IMAQ Rotate"("Use Bilinear Interpolation"=FALSE, "Maintain Size"=FALSE, "Angle (degrees)"=sgl 270.0, "Image Dst"=w1116, "Image Src"=w1116) -> ("Image Dst Out"=w1113:T4)  [unwired: 5 in, 1 out]
                                n448 = call "IMAQ Symmetry"("Type of Symmetry"=w1114, "Image Dst"=w1113, "Image Src"=w1113) -> ("Image Dst Out"=w1112:T4)  [unwired: 2 in, 1 out]
                                }
                                frame "Anticlockwise, No flip" {
                                n449 = call "IMAQ Rotate"("Use Bilinear Interpolation"=FALSE, "Maintain Size"=FALSE, "Angle (degrees)"=sgl 90.0, "Image Dst"=w1119, "Image Src"=w1119) -> ("Image Dst Out"=w1120:T4)  [unwired: 5 in, 1 out]
                                }
                                frame "Anticlockwise, Flip UD" {
                                w1126 = u32 0 items=["Horizontal", "Vertical", "Central", "1st Diagonal", "2nd Diagonal"] ("Type of Symmetry")
                                n450 = call "IMAQ Rotate"("Use Bilinear Interpolation"=FALSE, "Maintain Size"=FALSE, "Angle (degrees)"=sgl 90.0, "Image Dst"=w1128, "Image Src"=w1128) -> ("Image Dst Out"=w1125:T4)  [unwired: 5 in, 1 out]
                                n451 = call "IMAQ Symmetry"("Type of Symmetry"=w1126, "Image Dst"=w1125, "Image Src"=w1125) -> ("Image Dst Out"=w1124:T4)  [unwired: 2 in, 1 out]
                                }
                                frame "Anticlockwise, Flip LR" {
                                w1133 = u32 1 items=["Horizontal", "Vertical", "Central", "1st Diagonal", "2nd Diagonal"] ("Type of Symmetry")
                                n452 = call "IMAQ Rotate"("Use Bilinear Interpolation"=FALSE, "Maintain Size"=FALSE, "Angle (degrees)"=sgl 90.0, "Image Dst"=w1135, "Image Src"=w1135) -> ("Image Dst Out"=w1132:T4)  [unwired: 5 in, 1 out]
                                n453 = call "IMAQ Symmetry"("Type of Symmetry"=w1133, "Image Dst"=w1132, "Image Src"=w1132) -> ("Image Dst Out"=w1131:T4)  [unwired: 2 in, 1 out]
                                }
                                }
                                n454 = for {
                                tunnel: w1087 -> [w1090]
                                tunnel: w1085 -> [w1089] mode=indexing
                                tunnel: w1084 -> [w1088] mode=indexing
                                n455 = case shown="\"Camera 3\"" w1089 {
                                tunnel: w1090 -> [_ w1092]
                                tunnel: w1088 -> [_ w1091]
                                frame "None", Default {
                                }
                                frame "Camera 3" {
                                n456 = call "IMAQ Copy"("Image Dst"=w1091, "Image Src"=w1092) -> ()  [unwired: 4 in, 2 out]
                                }
                                }
                                }
                                }
                                frame 3 {
                                n457 = case shown="\"Anticlockwise, Flip UD\"" w1138 {
                                tunnel: w1139 -> [w1144 w1147 w1150 w1153 w1160 w1167 w1170 w1179 w1186]
                                tunnel: [w1144 w1146 w1149 w1151 w1156 w1163 w1171 w1175 w1182] -> w1140
                                frame "No rotation, No flip", Default {
                                }
                                frame "No rotation, Flip UD" {
                                w1145 = u32 0 items=["Horizontal", "Vertical", "Central", "1st Diagonal", "2nd Diagonal"] ("Type of Symmetry")
                                n458 = call "IMAQ Symmetry"("Type of Symmetry"=w1145, "Image Dst"=w1147, "Image Src"=w1147) -> ("Image Dst Out"=w1146:T4)  [unwired: 2 in, 1 out]
                                }
                                frame "No rotation, Flip LR" {
                                w1148 = u32 1 items=["Horizontal", "Vertical", "Central", "1st Diagonal", "2nd Diagonal"] ("Type of Symmetry")
                                n459 = call "IMAQ Symmetry"("Type of Symmetry"=w1148, "Image Dst"=w1150, "Image Src"=w1150) -> ("Image Dst Out"=w1149:T4)  [unwired: 2 in, 1 out]
                                }
                                frame "Clockwise, No flip" {
                                n460 = call "IMAQ Rotate"("Use Bilinear Interpolation"=FALSE, "Maintain Size"=FALSE, "Angle (degrees)"=sgl 270.0, "Image Dst"=w1153, "Image Src"=w1153) -> ("Image Dst Out"=w1151:T4)  [unwired: 5 in, 1 out]
                                }
                                frame "Clockwise, Flip UD" {
                                w1158 = u32 0 items=["Horizontal", "Vertical", "Central", "1st Diagonal", "2nd Diagonal"] ("Type of Symmetry")
                                n461 = call "IMAQ Rotate"("Use Bilinear Interpolation"=FALSE, "Maintain Size"=FALSE, "Angle (degrees)"=sgl 270.0, "Image Dst"=w1160, "Image Src"=w1160) -> ("Image Dst Out"=w1157:T4)  [unwired: 5 in, 1 out]
                                n462 = call "IMAQ Symmetry"("Type of Symmetry"=w1158, "Image Dst"=w1157, "Image Src"=w1157) -> ("Image Dst Out"=w1156:T4)  [unwired: 2 in, 1 out]
                                }
                                frame "Clockwise, Flip LR" {
                                w1165 = u32 1 items=["Horizontal", "Vertical", "Central", "1st Diagonal", "2nd Diagonal"] ("Type of Symmetry")
                                n463 = call "IMAQ Rotate"("Use Bilinear Interpolation"=FALSE, "Maintain Size"=FALSE, "Angle (degrees)"=sgl 270.0, "Image Dst"=w1167, "Image Src"=w1167) -> ("Image Dst Out"=w1164:T4)  [unwired: 5 in, 1 out]
                                n464 = call "IMAQ Symmetry"("Type of Symmetry"=w1165, "Image Dst"=w1164, "Image Src"=w1164) -> ("Image Dst Out"=w1163:T4)  [unwired: 2 in, 1 out]
                                }
                                frame "Anticlockwise, No flip" {
                                n465 = call "IMAQ Rotate"("Use Bilinear Interpolation"=FALSE, "Maintain Size"=FALSE, "Angle (degrees)"=sgl 90.0, "Image Dst"=w1170, "Image Src"=w1170) -> ("Image Dst Out"=w1171:T4)  [unwired: 5 in, 1 out]
                                }
                                frame "Anticlockwise, Flip UD" {
                                w1177 = u32 0 items=["Horizontal", "Vertical", "Central", "1st Diagonal", "2nd Diagonal"] ("Type of Symmetry")
                                n466 = call "IMAQ Rotate"("Use Bilinear Interpolation"=FALSE, "Maintain Size"=FALSE, "Angle (degrees)"=sgl 90.0, "Image Dst"=w1179, "Image Src"=w1179) -> ("Image Dst Out"=w1176:T4)  [unwired: 5 in, 1 out]
                                n467 = call "IMAQ Symmetry"("Type of Symmetry"=w1177, "Image Dst"=w1176, "Image Src"=w1176) -> ("Image Dst Out"=w1175:T4)  [unwired: 2 in, 1 out]
                                }
                                frame "Anticlockwise, Flip LR" {
                                w1184 = u32 1 items=["Horizontal", "Vertical", "Central", "1st Diagonal", "2nd Diagonal"] ("Type of Symmetry")
                                n468 = call "IMAQ Rotate"("Use Bilinear Interpolation"=FALSE, "Maintain Size"=FALSE, "Angle (degrees)"=sgl 90.0, "Image Dst"=w1186, "Image Src"=w1186) -> ("Image Dst Out"=w1183:T4)  [unwired: 5 in, 1 out]
                                n469 = call "IMAQ Symmetry"("Type of Symmetry"=w1184, "Image Dst"=w1183, "Image Src"=w1183) -> ("Image Dst Out"=w1182:T4)  [unwired: 2 in, 1 out]
                                }
                                }
                                n470 = call "IMAQ Copy"("Image Dst"=w1143, "Image Src"=w1140) -> ("Image Dst Out"=w1141:T4)  [unwired: 4 in, 1 out]
                                n471 = property class="ImageControl"(reference=w1142, "Value"=w1141) -> ()  [unwired: 1 in, 2 out]
                                }
                                }
                              }
                              frame True {
                              }
                            }
                            n472 = property class="Bool (strict)"(reference=w988) -> ("Value"=w991:bool)  [unwired: 1 in, 2 out]
                            n473 = Not(x=w991) -> (.not. x?=w990:bool)
                          }
                        }
                      }
                    }
                    frame True {
                    }
                  }
                  n474 = case shown="False" w912 {
                    tunnel: w911 -> [w1471 _]
                    tunnel: w919 -> [w1470 _]
                    tunnel: w915 -> [w1469 _]
                    tunnel: w872 -> [w1468 _]
                    tunnel: w891 -> [w1467 _]
                    tunnel: w892 -> [w1466 _]
                    tunnel: w893 -> [w1465 _]
                    tunnel: w894 -> [w1464 _]
                    tunnel: w888 -> [w1463 _]
                    tunnel: w885 -> [w1462 _]
                    tunnel: w881 -> [w1461 _]
                    tunnel: w880 -> [w1460 _]
                    tunnel: w879 -> [w1459 _]
                    tunnel: w878 -> [w1458 _]
                    tunnel: w895 -> [w1457 _]
                    tunnel: w906 -> [w1456 _]
                    tunnel: w876 -> [w1455 _]
                    tunnel: w882 -> [w1454 _]
                    tunnel: w877 -> [w1453 _]
                    tunnel: w902 -> [w1451 _]
                    frame False {
                      n475 = for {
                        N: w1468 -> [_]
                        tunnel: w1462 -> [w1492]
                        tunnel: w1460 -> [w1491]
                        tunnel: w1471 -> [w1490]
                        tunnel: w1469 -> [w1489]
                        tunnel: w1470 -> [w1488]
                        tunnel: w1461 -> [w1487]
                        tunnel: w1466 -> [w1485]
                        tunnel: w1467 -> [w1484]
                        tunnel: w1465 -> [w1483]
                        tunnel: w1464 -> [w1482]
                        tunnel: w1459 -> [w1481]
                        tunnel: w1463 -> [w1480]
                        tunnel: w1458 -> [w1479]
                        tunnel: w1457 -> [w1478]
                        tunnel: w1456 -> [w1477]
                        tunnel: w1455 -> [w1476]
                        border: u32 0 ("millisecond timer value") -> [_]
                        tunnel: w1454 -> [w1474]
                        tunnel: w1453 -> [w1473]
                        tunnel: w1451 -> [w1472]
                        stop <- w1475 stop-if-true
                        n476 = event shown="[1] <Session Out>: Frame Done" {
                          selector: w1490 -> [_ _]
                          dyn-events: _ -> [_ _]
                          timeout: 1000 -> [_ _]
                          tunnel: w1492 -> [_ _]
                          tunnel: w1491 -> [_ w1526]
                          tunnel: w1489 -> [_ w1520]
                          tunnel: w1488 -> [_ w1516]
                          tunnel: w1487 -> [_ w1519]
                          tunnel: w1485 -> [_ w1524]
                          tunnel: w1484 -> [_ w1496]
                          tunnel: w1483 -> [_ w1523]
                          tunnel: w1482 -> [_ w1522]
                          tunnel: w1481 -> [_ w1521]
                          tunnel: w1480 -> [_ w1517]
                          tunnel: w1479 -> [_ w1513]
                          tunnel: w1478 -> [_ w1518]
                          tunnel: w1477 -> [_ w1501]
                          tunnel: w1476 -> [w1495 w1512]
                          tunnel: [w1493 w1514] -> w1475
                          tunnel: w1474 -> [_ w1499]
                          tunnel: w1473 -> [_ w1498]
                          tunnel: w1472 -> [_ w1497]
                          event Timeout {
                            n477 = event-data() -> ()  [unwired: 1 in, 3 out]
                            n478 = property class="Bool (strict)"(reference=w1495) -> ("Value"=w1494:bool)  [unwired: 1 in, 2 out]
                            n479 = Not(x=w1494) -> (.not. x?=w1493:bool)
                          }
                          event event #0x0 {
                            # "Read data"
                            n480 = event-data() -> ()  [unwired: 1 in, 1 out]
                            n481 = Tick Count (ms)() -> (millisecond timer value=w1500:u32)
                            n482 = feedback #6() -> (w1509:u32)
                            n483 = call "Elapsed time.vi"("Start time (ms)"=w1509, "Current time (ms)"=w1500) -> ("Elapsed time"=w1511:u32)
                            n484 = Greater?(x=w1511, y=w1497) -> (0:w1505:bool)
                            n485 = Select(t=w1500, s=w1505, f=w1509) -> (s? t:f=w1510:u32)
                            n486 = feedback-in #6(w1510) -> ()
                            n487 = call <vilib>:"IMAQdx Get Image2.vi"("Buffer Number Mode (Next)"=IMAQdx_Buffer_Number_Mode."Last New", "Image In"=w1516, "Session In"=w1520) -> ("error out"=w1503:errorcluster, "Image Out"=w1504:T4)  [unwired: 5 in, 2 out]
                            n488 = Not A Number/Path/Refnum?(number/path/refnum=w1526) -> (NaN/Path/Refnum?=w1507:bool)
                            n489 = Not(x=w1505) -> (.not. x?=w1506:bool)
                            n490 = Or(x=w1507, y=w1506) -> (x .or. y?=w1508:bool)
                            n491 = case shown="\"'tiff'\", \"tif\"" w1496 {
                              tunnel: w1504 -> [w1528 w1572 w1575]
                              tunnel: w1524 -> [_ _ w1576]
                              tunnel: w1523 -> [w1529 _ _]
                              tunnel: w1522 -> [w1530 _ _]
                              tunnel: w1517 -> [w1534 _ _]
                              tunnel: w1513 -> [w1533 _ w1580]
                              tunnel: w1518 -> [w1532 _ w1577]
                              tunnel: w1503 -> [w1531 _ w1579]
                              tunnel: [w1527 w1572 w1575] -> w1502
                              frame "'tiff'", "tif" {
                                n492 = stacked-sequence {
                                tunnel: w1534 -> [_ w1548 _ _]
                                tunnel: w1533 -> [w1535 _ _ w1565]
                                tunnel: w1532 -> [_ _ w1563 _]
                                tunnel: w1531 -> [_ w1543 _ _]
                                tunnel: w1530 -> [_ w1542 _ _]
                                tunnel: w1529 -> [_ w1538 _ _]
                                tunnel: w1528 -> [_ w1540 w1554 _]
                                tunnel: [_ w1540 _ _] -> w1527
                                frame #0 {
                                n493 = call <vilib>:"Acquire Semaphore.vi"("semaphore"=w1535) -> ()  [unwired: 4 in, 3 out]
                                }
                                frame #1 {
                                n494 = Preview Queue Element(queue=w1538) -> (queue out=w1539:refnum<queue>, element=w1537:T11)  [unwired: 2 in, 2 out]
                                n495 = in-place {
                                in-place-border: w1540 -> [w1551]
                                in-place-border: w1543 -> [w1550]
                                n496 = in-place-dvr #7(w1542) -> ()  [unwired: 2 out]
                                n497 = call "IMAQ ImageToArray"("error in (no error)"=w1550, "Image"=w1551) -> ("Image Pixels (I16)"=w1549:i16[][])  [unwired: 2 in, 4 out]
                                n498 = in-place-dvr #7(w1549) -> (w1541:refnum<data-value>)  [unwired: 1 out]
                                }
                                n499 = Preview Queue Element(queue=w1548) -> (queue out=w1546:refnum<queue>, element=w1547:u32[])  [unwired: 2 in, 2 out]
                                n500 = call "TIFFStream Write.vi"("File data"=w1537, "Last image in file?"=FALSE, "Current and next IFD offset in"=w1547, "Image data reference"=w1541) -> ("Current and next IFD offset out"=w1545:u32[], "File data out"=w1536:T11)  [unwired: 5 in, 1 out]
                                n501 = Lossy Enqueue Element(queue=w1539, element=w1536) -> ()  [unwired: 1 in, 4 out]
                                n502 = Lossy Enqueue Element(queue=w1546, element=w1545) -> ()  [unwired: 1 in, 4 out]
                                }
                                frame #2 {
                                w1557 = u32 0
                                n503 = call "IMAQ Read Custom Data"("Key"="IMAQdxReceiveTimestampHigh", "Image"=w1554) -> ("Custom Data Out"=w1561:string, "Image (duplicate)"=w1560:T4)  [unwired: 7 in, 1 out]
                                n504 = Unflatten From String(type=w1557, binary string=w1561) -> (value=w1556:u32)  [unwired: 3 in, 2 out]
                                n505 = call "IMAQ Read Custom Data"("Key"="IMAQdxReceiveTimestampLow", "Image"=w1560) -> ("Custom Data Out"=w1558:string)  [unwired: 7 in, 2 out]
                                n506 = Unflatten From String(type=w1557, binary string=w1558) -> (value=w1555:u32)  [unwired: 3 in, 2 out]
                                n507 = Join Numbers(hi=w1556, lo=w1555) -> ((hi.lo)=w1552:u64)
                                n508 = Bundle("element"=enum16{"Camera 1", "Camera 2", "Camera 3"}."Camera 1", w1552) -> (w1553:T24)  [unwired: 1 in]
                                n509 = Enqueue Element(queue=w1563, element=w1553) -> ()  [unwired: 2 in, 3 out]
                                }
                                frame #3 {
                                n510 = call <vilib>:"Release Semaphore.vi"("semaphore"=w1565) -> ()  [unwired: 5 in, 2 out]
                                }
                                }
                              }
                              frame "None", Default {
                                w1568 = u32 0
                                n511 = call "IMAQ Read Custom Data"("Key"="IMAQdxReceiveTimestampHigh", "Image"=w1572) -> ("Custom Data Out"=w1573:string, "Image (duplicate)"=w1571:T4)  [unwired: 7 in, 1 out]
                                n512 = Unflatten From String(type=w1568, binary string=w1573) -> (value=w1567:u32)  [unwired: 3 in, 2 out]
                                n513 = call "IMAQ Read Custom Data"("Key"="IMAQdxReceiveTimestampLow", "Image"=w1571) -> ("Custom Data Out"=w1569:string)  [unwired: 7 in, 2 out]
                                n514 = Unflatten From String(type=w1568, binary string=w1569) -> (value=w1566:u32)  [unwired: 3 in, 2 out]
                                n515 = Join Numbers(hi=w1567, lo=w1566) -> ()  [unwired: 1 out]
                              }
                              frame "dat", "u16" {
                                n516 = call "IMAQ ImageToArray"("error in (no error)"=w1579, "Image"=w1575) -> ("Image Pixels (I16)"=w1578:i16[][])  [unwired: 2 in, 4 out]
                                n517 = stacked-sequence {
                                seq-local: [_ _ w1585 _ _] -> [_ _ _ w1595 _]
                                tunnel: w1578 -> [_ w1583 _ _ _]
                                tunnel: w1576 -> [_ w1582 _ _ _]
                                tunnel: w1580 -> [w1581 _ _ _ w1599]
                                tunnel: w1577 -> [_ _ _ w1598 _]
                                tunnel: w1575 -> [_ _ w1586 _ _]
                                frame #0 {
                                n518 = call <vilib>:"Acquire Semaphore.vi"("semaphore"=w1581) -> ()  [unwired: 4 in, 3 out]
                                }
                                frame #1 {
                                n519 = Write to Binary File(file (use dialog)=w1582, data=w1583, 5:FALSE ("prepend array or string size? (T)")) -> ()  [unwired: 3 in, 3 out]
                                }
                                frame #2 {
                                w1589 = u32 0
                                n520 = call "IMAQ Read Custom Data"("Key"="IMAQdxReceiveTimestampHigh", "Image"=w1586) -> ("Custom Data Out"=w1593:string, "Image (duplicate)"=w1592:T4)  [unwired: 7 in, 1 out]
                                n521 = Unflatten From String(type=w1589, binary string=w1593) -> (value=w1588:u32)  [unwired: 3 in, 2 out]
                                n522 = call "IMAQ Read Custom Data"("Key"="IMAQdxReceiveTimestampLow", "Image"=w1592) -> ("Custom Data Out"=w1590:string)  [unwired: 7 in, 2 out]
                                n523 = Unflatten From String(type=w1589, binary string=w1590) -> (value=w1587:u32)  [unwired: 3 in, 2 out]
                                n524 = Join Numbers(hi=w1588, lo=w1587) -> ((hi.lo)=w1585:u64)
                                }
                                frame #3 {
                                n525 = Bundle("element"=enum16{"Camera 1", "Camera 2", "Camera 3"}."Camera 1", w1595) -> (w1597:T24)  [unwired: 1 in]
                                n526 = Enqueue Element(queue=w1598, element=w1597) -> ()  [unwired: 2 in, 3 out]
                                }
                                frame #4 {
                                n527 = call <vilib>:"Release Semaphore.vi"("semaphore"=w1599) -> ()  [unwired: 5 in, 2 out]
                                }
                                }
                              }
                            }
                            n528 = case shown="False" w1508 {
                              tunnel: w1526 -> [w1605 _]
                              tunnel: w1519 -> [w1606 _]
                              tunnel: w1521 -> [w1604 _]
                              tunnel: w1502 -> [w1603 _]
                              tunnel: w1501 -> [w1600 _]
                              tunnel: w1499 -> [w1602 _]
                              tunnel: w1498 -> [w1601 _]
                              frame False {
                                n529 = case shown="1" w1606 {
                                tunnel: w1605 -> [_ _ w1667]
                                tunnel: w1604 -> [_ _ w1666]
                                tunnel: w1603 -> [_ w1610 w1663]
                                tunnel: w1602 -> [_ w1609 _]
                                tunnel: w1601 -> [_ w1608 _]
                                tunnel: w1600 -> [_ w1607 w1662]
                                frame -1, Default {
                                }
                                frame 0 {
                                n530 = case shown="\"Anticlockwise, Flip UD\"" w1607 {
                                tunnel: w1610 -> [w1617 w1620 w1623 w1626 w1633 w1640 w1643 w1652 w1659]
                                tunnel: [w1617 w1619 w1622 w1624 w1629 w1636 w1644 w1648 w1655] -> w1611
                                frame "No rotation, No flip", Default {
                                }
                                frame "No rotation, Flip UD" {
                                w1618 = u32 0 items=["Horizontal", "Vertical", "Central", "1st Diagonal", "2nd Diagonal"] ("Type of Symmetry")
                                n531 = call "IMAQ Symmetry"("Type of Symmetry"=w1618, "Image Dst"=w1620, "Image Src"=w1620) -> ("Image Dst Out"=w1619:T4)  [unwired: 2 in, 1 out]
                                }
                                frame "No rotation, Flip LR" {
                                w1621 = u32 1 items=["Horizontal", "Vertical", "Central", "1st Diagonal", "2nd Diagonal"] ("Type of Symmetry")
                                n532 = call "IMAQ Symmetry"("Type of Symmetry"=w1621, "Image Dst"=w1623, "Image Src"=w1623) -> ("Image Dst Out"=w1622:T4)  [unwired: 2 in, 1 out]
                                }
                                frame "Clockwise, No flip" {
                                n533 = call "IMAQ Rotate"("Use Bilinear Interpolation"=FALSE, "Maintain Size"=FALSE, "Angle (degrees)"=sgl 270.0, "Image Dst"=w1626, "Image Src"=w1626) -> ("Image Dst Out"=w1624:T4)  [unwired: 5 in, 1 out]
                                }
                                frame "Clockwise, Flip UD" {
                                w1631 = u32 0 items=["Horizontal", "Vertical", "Central", "1st Diagonal", "2nd Diagonal"] ("Type of Symmetry")
                                n534 = call "IMAQ Rotate"("Use Bilinear Interpolation"=FALSE, "Maintain Size"=FALSE, "Angle (degrees)"=sgl 270.0, "Image Dst"=w1633, "Image Src"=w1633) -> ("Image Dst Out"=w1630:T4)  [unwired: 5 in, 1 out]
                                n535 = call "IMAQ Symmetry"("Type of Symmetry"=w1631, "Image Dst"=w1630, "Image Src"=w1630) -> ("Image Dst Out"=w1629:T4)  [unwired: 2 in, 1 out]
                                }
                                frame "Clockwise, Flip LR" {
                                w1638 = u32 1 items=["Horizontal", "Vertical", "Central", "1st Diagonal", "2nd Diagonal"] ("Type of Symmetry")
                                n536 = call "IMAQ Rotate"("Use Bilinear Interpolation"=FALSE, "Maintain Size"=FALSE, "Angle (degrees)"=sgl 270.0, "Image Dst"=w1640, "Image Src"=w1640) -> ("Image Dst Out"=w1637:T4)  [unwired: 5 in, 1 out]
                                n537 = call "IMAQ Symmetry"("Type of Symmetry"=w1638, "Image Dst"=w1637, "Image Src"=w1637) -> ("Image Dst Out"=w1636:T4)  [unwired: 2 in, 1 out]
                                }
                                frame "Anticlockwise, No flip" {
                                n538 = call "IMAQ Rotate"("Use Bilinear Interpolation"=FALSE, "Maintain Size"=FALSE, "Angle (degrees)"=sgl 90.0, "Image Dst"=w1643, "Image Src"=w1643) -> ("Image Dst Out"=w1644:T4)  [unwired: 5 in, 1 out]
                                }
                                frame "Anticlockwise, Flip UD" {
                                w1650 = u32 0 items=["Horizontal", "Vertical", "Central", "1st Diagonal", "2nd Diagonal"] ("Type of Symmetry")
                                n539 = call "IMAQ Rotate"("Use Bilinear Interpolation"=FALSE, "Maintain Size"=FALSE, "Angle (degrees)"=sgl 90.0, "Image Dst"=w1652, "Image Src"=w1652) -> ("Image Dst Out"=w1649:T4)  [unwired: 5 in, 1 out]
                                n540 = call "IMAQ Symmetry"("Type of Symmetry"=w1650, "Image Dst"=w1649, "Image Src"=w1649) -> ("Image Dst Out"=w1648:T4)  [unwired: 2 in, 1 out]
                                }
                                frame "Anticlockwise, Flip LR" {
                                w1657 = u32 1 items=["Horizontal", "Vertical", "Central", "1st Diagonal", "2nd Diagonal"] ("Type of Symmetry")
                                n541 = call "IMAQ Rotate"("Use Bilinear Interpolation"=FALSE, "Maintain Size"=FALSE, "Angle (degrees)"=sgl 90.0, "Image Dst"=w1659, "Image Src"=w1659) -> ("Image Dst Out"=w1656:T4)  [unwired: 5 in, 1 out]
                                n542 = call "IMAQ Symmetry"("Type of Symmetry"=w1657, "Image Dst"=w1656, "Image Src"=w1656) -> ("Image Dst Out"=w1655:T4)  [unwired: 2 in, 1 out]
                                }
                                }
                                n543 = for {
                                tunnel: w1611 -> [w1614]
                                tunnel: w1609 -> [w1613] mode=indexing
                                tunnel: w1608 -> [w1612] mode=indexing
                                n544 = case shown="\"Camera 1\"" w1613 {
                                tunnel: w1614 -> [_ w1616]
                                tunnel: w1612 -> [_ w1615]
                                frame "None", Default {
                                }
                                frame "Camera 1" {
                                n545 = call "IMAQ Copy"("Image Dst"=w1615, "Image Src"=w1616) -> ()  [unwired: 4 in, 2 out]
                                }
                                }
                                }
                                }
                                frame 1 {
                                n546 = case shown="\"Anticlockwise, Flip UD\"" w1662 {
                                tunnel: w1663 -> [w1668 w1671 w1674 w1677 w1684 w1691 w1694 w1703 w1710]
                                tunnel: [w1668 w1670 w1673 w1675 w1680 w1687 w1695 w1699 w1706] -> w1664
                                frame "No rotation, No flip", Default {
                                }
                                frame "No rotation, Flip UD" {
                                w1669 = u32 0 items=["Horizontal", "Vertical", "Central", "1st Diagonal", "2nd Diagonal"] ("Type of Symmetry")
                                n547 = call "IMAQ Symmetry"("Type of Symmetry"=w1669, "Image Dst"=w1671, "Image Src"=w1671) -> ("Image Dst Out"=w1670:T4)  [unwired: 2 in, 1 out]
                                }
                                frame "No rotation, Flip LR" {
                                w1672 = u32 1 items=["Horizontal", "Vertical", "Central", "1st Diagonal", "2nd Diagonal"] ("Type of Symmetry")
                                n548 = call "IMAQ Symmetry"("Type of Symmetry"=w1672, "Image Dst"=w1674, "Image Src"=w1674) -> ("Image Dst Out"=w1673:T4)  [unwired: 2 in, 1 out]
                                }
                                frame "Clockwise, No flip" {
                                n549 = call "IMAQ Rotate"("Use Bilinear Interpolation"=FALSE, "Maintain Size"=FALSE, "Angle (degrees)"=sgl 270.0, "Image Dst"=w1677, "Image Src"=w1677) -> ("Image Dst Out"=w1675:T4)  [unwired: 5 in, 1 out]
                                }
                                frame "Clockwise, Flip UD" {
                                w1682 = u32 0 items=["Horizontal", "Vertical", "Central", "1st Diagonal", "2nd Diagonal"] ("Type of Symmetry")
                                n550 = call "IMAQ Rotate"("Use Bilinear Interpolation"=FALSE, "Maintain Size"=FALSE, "Angle (degrees)"=sgl 270.0, "Image Dst"=w1684, "Image Src"=w1684) -> ("Image Dst Out"=w1681:T4)  [unwired: 5 in, 1 out]
                                n551 = call "IMAQ Symmetry"("Type of Symmetry"=w1682, "Image Dst"=w1681, "Image Src"=w1681) -> ("Image Dst Out"=w1680:T4)  [unwired: 2 in, 1 out]
                                }
                                frame "Clockwise, Flip LR" {
                                w1689 = u32 1 items=["Horizontal", "Vertical", "Central", "1st Diagonal", "2nd Diagonal"] ("Type of Symmetry")
                                n552 = call "IMAQ Rotate"("Use Bilinear Interpolation"=FALSE, "Maintain Size"=FALSE, "Angle (degrees)"=sgl 270.0, "Image Dst"=w1691, "Image Src"=w1691) -> ("Image Dst Out"=w1688:T4)  [unwired: 5 in, 1 out]
                                n553 = call "IMAQ Symmetry"("Type of Symmetry"=w1689, "Image Dst"=w1688, "Image Src"=w1688) -> ("Image Dst Out"=w1687:T4)  [unwired: 2 in, 1 out]
                                }
                                frame "Anticlockwise, No flip" {
                                n554 = call "IMAQ Rotate"("Use Bilinear Interpolation"=FALSE, "Maintain Size"=FALSE, "Angle (degrees)"=sgl 90.0, "Image Dst"=w1694, "Image Src"=w1694) -> ("Image Dst Out"=w1695:T4)  [unwired: 5 in, 1 out]
                                }
                                frame "Anticlockwise, Flip UD" {
                                w1701 = u32 0 items=["Horizontal", "Vertical", "Central", "1st Diagonal", "2nd Diagonal"] ("Type of Symmetry")
                                n555 = call "IMAQ Rotate"("Use Bilinear Interpolation"=FALSE, "Maintain Size"=FALSE, "Angle (degrees)"=sgl 90.0, "Image Dst"=w1703, "Image Src"=w1703) -> ("Image Dst Out"=w1700:T4)  [unwired: 5 in, 1 out]
                                n556 = call "IMAQ Symmetry"("Type of Symmetry"=w1701, "Image Dst"=w1700, "Image Src"=w1700) -> ("Image Dst Out"=w1699:T4)  [unwired: 2 in, 1 out]
                                }
                                frame "Anticlockwise, Flip LR" {
                                w1708 = u32 1 items=["Horizontal", "Vertical", "Central", "1st Diagonal", "2nd Diagonal"] ("Type of Symmetry")
                                n557 = call "IMAQ Rotate"("Use Bilinear Interpolation"=FALSE, "Maintain Size"=FALSE, "Angle (degrees)"=sgl 90.0, "Image Dst"=w1710, "Image Src"=w1710) -> ("Image Dst Out"=w1707:T4)  [unwired: 5 in, 1 out]
                                n558 = call "IMAQ Symmetry"("Type of Symmetry"=w1708, "Image Dst"=w1707, "Image Src"=w1707) -> ("Image Dst Out"=w1706:T4)  [unwired: 2 in, 1 out]
                                }
                                }
                                n559 = call "IMAQ Copy"("Image Dst"=w1667, "Image Src"=w1664) -> ("Image Dst Out"=w1665:T4)  [unwired: 4 in, 1 out]
                                n560 = property class="ImageControl"(reference=w1666, "Value"=w1665) -> ()  [unwired: 1 in, 2 out]
                                }
                                }
                              }
                              frame True {
                              }
                            }
                            n561 = property class="Bool (strict)"(reference=w1512) -> ("Value"=w1515:bool)  [unwired: 1 in, 2 out]
                            n562 = Not(x=w1515) -> (.not. x?=w1514:bool)
                          }
                        }
                      }
                    }
                    frame True {
                    }
                  }
                }
                frame #1 {
                  n563 = Send Notification(notification=TRUE, notifier=w1714) -> ()  [unwired: 1 in, 2 out]
                }
              }
              n564 = node-c288(w746, 10 ("Priority")) -> (w766:T13)  [unwired: 2 in]
              n565 = timed-loop {
                timing: w766 -> [_]
                timing-out: [_] -> w765
                tunnel: w764 -> [w787]
                tunnel: w760 -> [w785]
                tunnel: w758 -> [w784]
                tunnel: w757 -> [_]
                stop <- w786 stop-if-true
                n566 = node-c288() -> ()  [unwired: 1 in, 1 out]
                n567 = Get Notifier Status(notifier=w787) -> (current notification=w786:bool)  [unwired: 1 in, 4 out]
                n568 = Unbundle By Name(w785) -> ("Offset and gain"=w780:dbl[][], "RGB Channels"=w783:T19, "RGB buffers"=w782:T4[], "Current camera"=w781:i32)
                n569 = case shown="0" w781 {
                  tunnel: w780 -> [_ w814]
                  tunnel: w783 -> [_ w813]
                  tunnel: w782 -> [_ w788]
                  tunnel: w784 -> [_ w810]
                  frame 1, Default {
                  }
                  frame 0 {
                    w798 = 0 ("X Resolution")
                    w801 = u16 0 items=["RGB", "HSL", "HSV", "HSI"] ("Color Mode")
                    n570 = Index Array(array=w788, index #1=0 ("index"), index #2=1 ("index")) -> (element #1=w795:T4, element #2=w808:T4)
                    n571 = Array Subset(array=w788, index=2 ("length"), length=3 ("index")) -> (w812:T4[])
                    n572 = Array Subset(array=w788, index=5 ("length"), length=3 ("index")) -> (w789:T4[])
                    n573 = for {
                      tunnel: w812 -> [w828] mode=indexing
                      tunnel: w814 -> [w827] mode=indexing
                      tunnel: w813 -> [w829] mode=indexing
                      tunnel: [w826] -> w807 mode=indexing
                      tunnel: w808 -> [w825]
                      shift-right: [w821] -> w797
                      shift-left: w798 -> [w824]
                      shift-right: [w822] -> w796
                      shift-left: w798 -> [w823]
                      tunnel: w795 -> [w820]
                      tunnel: w789 -> [w819] mode=indexing
                      n574 = case shown="\"Camera 1\", Default" w829 {
                        tunnel: w828 -> [w833 w850]
                        tunnel: w827 -> [_ w860]
                        tunnel: [w839 w849] -> w826
                        tunnel: w825 -> [_ w862]
                        tunnel: w824 -> [w837 w846]
                        tunnel: w823 -> [w835 w844]
                        tunnel: [w835 w843] -> w822
                        tunnel: [w837 w842] -> w821
                        tunnel: w820 -> [w838 _]
                        tunnel: w819 -> [_ w841]
                        frame "None" {
                          n575 = call "IMAQ GetImageSize"("Image"=w838) -> ("Y Resolution"=w834:i32, "X Resolution"=w836:i32)  [unwired: 3 in, 1 out]
                          n576 = Max & Min(x=w837, y=w836) -> (max(x,y)=w831:i32)  [unwired: 1 out]
                          n577 = Max & Min(x=w835, y=w834) -> (max(x,y)=w830:i32)  [unwired: 1 out]
                          n578 = call "IMAQ SetImageSize"("Y Resolution"=w830, "X Resolution"=w831, "Image"=w833) -> ("Image Out"=w832:T4)  [unwired: 2 in, 1 out]
                          n579 = call "IMAQ FillImage"("Pixel Value (U8, U16, I16, Float)"=sgl 0.0, "Image"=w832) -> ("Image Out"=w839:T4)  [unwired: 8 in, 1 out]
                        }
                        frame "Camera 1", Default {
                          w851 = T17 0 items=["Grayscale (U8)", "Grayscale (I16)", "Grayscale (SGL)", "Complex (CSG)", "RGB (U32)", "HSL (U32)", "RGB (U64)", "Grayscale (U16)"] ("Image Type")
                          w861 = T17 2 items=["Grayscale (U8)", "Grayscale (I16)", "Grayscale (SGL)", "Complex (CSG)", "RGB (U32)", "HSL (U32)", "RGB (U64)", "Grayscale (U16)"] ("Image Type")
                          n580 = call "IMAQ GetImageSize"("Image"=w841) -> ("Y Resolution"=w845:i32, "X Resolution"=w847:i32, "error out"=w848:errorcluster)  [unwired: 3 in]
                          n581 = Index Array(array=w860, index #1=0 ("index"), index #2=1 ("index")) -> (element #1=w857:dbl, element #2=w853:dbl)
                          n582 = call "IMAQ Cast Image"("Image Type"=w861, "error in (no error)"=w848, "Image Dst"=w862, "Image Src"=w841) -> ("Image Dst Out"=w856:T4)  [unwired: 6 in, 1 out]
                          n583 = Max & Min(x=w846, y=w847) -> (max(x,y)=w842:i32)  [unwired: 1 out]
                          n584 = Max & Min(x=w844, y=w845) -> (max(x,y)=w843:i32)  [unwired: 1 out]
                          n585 = call "IMAQ Add"("Image Src A"=w856, "Constant"=w857, "Image Dst"=w856) -> ("Image Dst Out"=w854:T4, "error out"=w855:errorcluster)  [unwired: 4 in]
                          n586 = call "IMAQ Multiply"("Image Src A"=w854, "Constant"=w853, "Image Dst"=w854, "error in (no error)"=w855) -> ("Image Dst Out"=w852:T4)  [unwired: 3 in, 1 out]
                          n587 = call "IMAQ Cast Image"("Image Type"=w851, "Image Dst"=w850, "Image Src"=w852) -> ("Image Dst Out"=w849:T4)  [unwired: 7 in, 1 out]
                        }
                      }
                    }
                    n588 = Index Array(array=w807, index #1=0 ("index"), index #2=1 ("index"), index #3=2 ("index")) -> (element #1=w799:T4, element #2=w803:T4, element #3=w802:T4)
                    n589 = call "IMAQ SetImageSize"("Y Resolution"=w796, "X Resolution"=w797, "Image"=w795) -> ("error out"=w793:errorcluster, "Image Out"=w800:T4)  [unwired: 2 in]
                    n590 = call "IMAQ ReplaceColorPlane"("Image Src"=w800, "Color Mode"=w801, "Image Dst"=w800, "Red or Hue Plane"=w799, "Green or Sat Plane"=w803, "error in (no error)"=w793, "Blue or Luma or Val or Inten Plane"=w802) -> ("Image Dst Out"=w794:T4, "error out"=w792:errorcluster)  [unwired: 7 in]
                    n591 = case shown="No Error" w792 {
                      tunnel: w810 -> [w818 _]
                      tunnel: w794 -> [w817 _]
                      frame No Error {
                        n592 = property class="ImageControl"(reference=w818, "Value"=w817) -> ()  [unwired: 1 in, 2 out]
                      }
                      frame Error {
                      }
                    }
                  }
                }
                n593 = node-c288() -> ()  [unwired: 1 in, 1 out]
              }
              n594 = node-c288(w765) -> ()  [unwired: 1 out]
            }
            frame #3 {
              n595 = disable-structure shown="Enabled" {
                disable-tunnel: w1722 -> [_ w1774]
                frame Disabled {
                }
                frame Enabled {
                  n596 = for {
                    tunnel: w1774 -> [w1776] mode=indexing
                    n597 = call <vilib>:"IMAQdx Stop Acquisition.vi"("Session In"=w1776) -> ("Session Out"=w1775:T3)  [unwired: 9 in, 1 out]
                    n598 = call <vilib>:"IMAQdx Unconfigure Acquisition.vi"("Session In"=w1775) -> ()  [unwired: 9 in, 2 out]
                  }
                }
              }
              n599 = case shown="\"dat\", \"u16\"" w1721 {
                tunnel: w1720 -> [_ _ w1764]
                tunnel: w1719 -> [w1725 _ _]
                tunnel: w1718 -> [w1741 _ _]
                tunnel: w1717 -> [w1729 _ w1756]
                tunnel: w1716 -> [w1736 _ w1763]
                tunnel: w1715 -> [w1735 _ _]
                frame "'tiff'", "tif" {
                  n600 = Dequeue Element(queue=w1725) -> (queue out=w1723:refnum<queue>, element=w1724:T11)  [unwired: 2 in, 2 out]
                  n601 = Flush Queue(queue=w1729) -> (queue out=w1733:refnum<queue>, remaining elements=w1732:T25, error out=w1731:errorcluster)  [unwired: 1 in]
                  n602 = Preview Queue Element(queue=w1735) -> (element=w1734:u32[])  [unwired: 2 in, 3 out]
                  n603 = call "TIFFStream Close.vi"("Current and next IFD offset"=w1734, "Image data reference"=w1741, "File data"=w1724) -> ()  [unwired: 8 in, 1 out]
                  n604 = Release Queue(queue=w1723) -> ()  [unwired: 2 in, 3 out]
                  n605 = for {
                    tunnel: w1732 -> [w1750] mode=indexing
                    tunnel: [w1749] -> w1730 mode=indexing
                    n606 = Unbundle(w1750) -> ("Camera identity"=w1747:enum16{"Camera 1", "Camera 2", "Camera 3"}, "Timestamp"=w1748:u64)
                    n607 = Increment(x=w1747) -> (x+1=w1742:enum16{"Camera 1", "Camera 2", "Camera 3"})
                    n608 = Number To Decimal String(number=w1748) -> (decimal integer string=w1745:string)  [unwired: 1 in]
                    n609 = Number To Decimal String(number=w1742) -> (decimal integer string=w1746:string)  [unwired: 1 in]
                    n610 = call <vilib>:"Space Constant.vi"() -> ("String"=w1744:string)
                    n611 = Concatenate Strings(w1746, w1744, w1745, "\r") -> (w1749:string)
                  }
                  n612 = Release Queue(queue=w1733, error in (no error)=w1731) -> ()  [unwired: 1 in, 3 out]
                  n613 = Strip Path(path=w1736) -> (stripped path=w1740:path)  [unwired: 1 out]
                  n614 = call <vilib>:"Get File Extension.vi"("file"=w1736) -> ("filename without extension"=w1738:string)  [unwired: 6 in, 4 out]
                  n615 = Concatenate Strings(w1738, "_FrameOrder.txt" ("string")) -> (w1739:string)
                  n616 = Build Path(base path=w1740, name or relative path=w1739) -> (appended path=w1728:path)
                  n617 = Concatenate Strings(w1730) -> (w1727:string)
                  n618 = Write to Text File(file (use dialog)=w1728, text=w1727) -> (refnum out=w1726:refnum<file>)  [unwired: 2 in, 2 out]
                  n619 = Close File(refnum=w1726) -> ()  [unwired: 1 in, 2 out]
                }
                frame "None", Default {
                }
                frame "dat", "u16" {
                  n620 = Close File(refnum=w1764) -> ()  [unwired: 1 in, 2 out]
                  n621 = Flush Queue(queue=w1756) -> (queue out=w1757:refnum<queue>, remaining elements=w1752:T25, error out=w1755:errorcluster)  [unwired: 1 in]
                  n622 = Strip Path(path=w1763) -> (stripped path=w1762:path)  [unwired: 1 out]
                  n623 = call <vilib>:"Get File Extension.vi"("file"=w1763) -> ("filename without extension"=w1760:string)  [unwired: 6 in, 4 out]
                  n624 = Concatenate Strings(w1760, "_FrameOrder.txt" ("string")) -> (w1761:string)
                  n625 = Release Queue(queue=w1757, error in (no error)=w1755) -> ()  [unwired: 1 in, 3 out]
                  n626 = for {
                    tunnel: w1752 -> [w1773] mode=indexing
                    tunnel: [w1772] -> w1753 mode=indexing
                    n627 = Unbundle(w1773) -> ("Camera identity"=w1770:enum16{"Camera 1", "Camera 2", "Camera 3"}, "Timestamp"=w1771:u64)
                    n628 = Increment(x=w1770) -> (x+1=w1765:enum16{"Camera 1", "Camera 2", "Camera 3"})
                    n629 = Number To Decimal String(number=w1771) -> (decimal integer string=w1768:string)  [unwired: 1 in]
                    n630 = Number To Decimal String(number=w1765) -> (decimal integer string=w1769:string)  [unwired: 1 in]
                    n631 = call <vilib>:"Space Constant.vi"() -> ("String"=w1767:string)
                    n632 = Concatenate Strings(w1769, w1767, w1768, "\r") -> (w1772:string)
                  }
                  n633 = Build Path(base path=w1762, name or relative path=w1761) -> (appended path=w1758:path)
                  n634 = Concatenate Strings(w1753) -> (w1751:string)
                  n635 = Write to Text File(file (use dialog)=w1758, text=w1751) -> (refnum out=w1754:refnum<file>)  [unwired: 2 in, 2 out]
                  n636 = Close File(refnum=w1754) -> ()  [unwired: 1 in, 2 out]
                }
              }
            }
          }
        }
      }
    }
    frame "Get status" {
      n637 = Variant To Data(type=w1786, Variant=w1787) -> (data=w1785:T6)  [unwired: 1 in, 1 out]
      n638 = Unbundle By Name(w1785) -> ("Camera References"=w1784:T3[], "Current camera"=w1783:i32)
      n639 = Decrement(x=w1783) -> (x-1=w1779:i32)
      n640 = Max & Min(x=w1779, y=1) -> (max(x,y)=w1777:i32)  [unwired: 1 out]
      n641 = Index Array(array=w1784, index=w1777) -> (element=w1782:T3)
      n642 = property class="IMAQdx"(reference=w1782, "ActiveAttribute"="CameraAttributes::DeviceControl::DeviceTemperature") -> (error out=w1781:errorcluster, "ValueDBL"=w1788:dbl)  [unwired: 1 in, 1 out]
      n643 = Unbundle By Name(w1781) -> ("status"=w1780:bool)
      n644 = Bundle By Name(cluster=w1791, "System OK?"=w1780, "Temperature"=w1788) -> (w1790:T1)
    }
    frame "Other settings" {
      n645 = Variant To Data(type=w1807, Variant=w1808) -> (data=w1803:T6)  [unwired: 1 in, 1 out]
      n646 = Unbundle By Name(w1803) -> ("Offset and gain"=w1794:dbl[][], "Camera References"=w1806:T3[], "Current camera"=w1805:i32, "Which cameras record"=w1804:bool[], "RGB Channels"=w1796:T19, "Image buffers"=w1795:T4[], "Camera orientation"=w1793:T18)
      n647 = call "PointGrey Grasshopper_Settings.vi"("Camera References"=w1806, "Offset and gain"=w1794, "Camera to address"=w1805, "Camera orientation"=w1793, "Which cameras record"=w1804, "RGB Channels in"=w1796, "Image buffers"=w1795) -> ("Offset gain out"=w1798:dbl[][], "Camera to address out"=w1799:i32, "Camera orientation out"=w1792:T18, "Which cameras record out"=w1802:bool[], "RGB Channels out"=w1797:T19)  [unwired: 4 in]
      n648 = Bundle By Name(cluster=w1803, "Offset and gain"=w1798, "Current camera"=w1799, "Which cameras record"=w1802, "RGB Channels"=w1797, "Camera orientation"=w1792) -> (w1800:T6)
      n649 = To Variant(anything=w1800) -> (Variant=w1801:variant)
    }
  }
  "Status" <- w8
  "Camera-specific out" <- w5
